vi "SISE-Monitor100.vi"() -> ()   [LabVIEW 2024]
uses:
  SubVIs-SISE-Monitor100/Control-IonFlux.ctl
  <vilib>/DAQmx/read.llb/DAQmx Read (Analog 2D DBL NChan NSamp).vi
  <vilib>/Instr/_visa.llb/VISA Configure Serial Port (Instr).vi
  <vilib>/DAQmx/create/channels.llb/DAQmx Create Channel (AI-Voltage-Basic).vi
  <vilib>/DAQmx/miscellaneous.llb/DAQmx Fill In Error Info.vi
  <vilib>/Analysis/NI_AALPro.lvlib
panel:
  out "Lesepuffer":string
  out "Registerkarte":enum32{"Start", "Record", "Stop"}(tab)
  out "Output V ch 2":bool
  in  "V channel 2":bool
  out "Output V ch 1":bool
  in  "V channel 1":bool
  out "SISE channel 1":bool
  out "Output SISE ch 2":bool
  in  "SISE channel 2":bool
  out "slow":bool
  in  "Scan angle (degrees)":dbl(slide) scale=0.0..90.0
  out "?":dbl
  in  "VISA res. name":refnum<visa-resource-name> caption="VISA-Ressourcenname"
  in  "Start measurement":bool
  out "Data File":bool
  out "Ind. Channel In":bool
  in  "Data file":path
  out "Ind. Channel Out":bool
  out "?":dbl
  out "Record period (round at 5s)":dbl
  in  "Scan distance (µm)":dbl(slide)=50.0 scale=0.0..100.0
  in  "Record period (single track, s)":dbl(slide)=10.112359550561797 scale=0.0..60.0 scale format="%#_2f"
  in  "Manipulator Speed":bool
  out "fast":bool
  in  "Channels In":tag
  in  "Position of manipulator":bool
  out "right":bool
  out "left":bool
  in  "TC 3":T1(tab)
  in  "Range limit\nS1.1 (mV)":dbl(slide)=200.0 min=0.0 max=600.0 scale=0.2..600.0
  in  "Base line\nS1.1 (mV)":dbl(slide) scale=-300.0..300.0
  in  "Range limit\nS1.2 mV":dbl(slide)=30.0 scale=0.1..30.0
  in  "Base line \nS1.2 (mV)":dbl(slide) scale=-15.0..15.0
  out "dV-SISE channel 1":cluster{dbl[], dbl[]}[](graph)
  out "V-SISE channel 1":cluster{dbl[], dbl[]}[](graph)
  out "V-SISE channel 2":cluster{dbl[], dbl[]}[](graph)
  out "dV-SISE channel 2":cluster{dbl[], dbl[]}[](graph)
  in  "Range limit\nS2.1 (mV)":dbl(slide)=200.0 min=0.0 max=600.0 scale=0.2..600.0
  in  "Base line\nS2.1 (mV)":dbl(slide) scale=-300.0..300.0
  in  "Base line \nS2.2 (mV)":dbl(slide) scale=-15.0..15.0
  in  "Range limit\nS2.2 (mV)":dbl(slide)=30.0 scale=0.1..30.0
  out "Voltage channel 1":cluster{dbl[], dbl[]}[](graph)
  in  "Base line\nV1 (V)":dbl(slide) scale=-10.0..10.0
  in  "Range limit\nV1 (V)":dbl(slide)=24.63054187192118 min=0.0 max=600.0 scale=0.0..25.0
  in  "Base line\nV2 (V)":dbl(slide) scale=-10.0..10.0
  in  "Range limit\nV2 (V)":dbl(slide)=24.63054187192118 min=0.0 max=600.0 scale=0.0..25.0
  out "Voltage channel 2":cluster{dbl[], dbl[]}[](graph)
  out "V channel #2":bool
  out "V channel #1":bool
  out "SISE channel #2":bool
  out "SISE channel #1":bool
  in  "?":T2(tab)
  out "Vprobe SISE 1":cluster{dbl[], dbl[]}[](graph)
  out "Vprobe SISE 2":cluster{dbl[], dbl[]}[](graph)
  out "Vprobe V 1":cluster{dbl[], dbl[]}[](graph)
  out "Vprobe V 2":cluster{dbl[], dbl[]}[](graph)
  in  "Enable change position 0":bool
  out "Raw data file":path
  in  "Stop measurent":bool
  out "Position probe":cluster{dbl[], dbl[]}[](graph)
  in  "Add Mark":bool
  in  "Event Mark":string
  out "Stop recording":bool
  out "String":string
  out "E-mark on":T3
  out "?":string
  in  "Bildlaufleiste":i32(c297)
  in  "Start fit (% of rec. period)":dbl(slide)=50.0 scale=0.0..100.0
  in  "?":enum32{"dV SISE 1", "dV SISE 2"}(tab)
  out "deltaV SISE 1":cluster{dbl[], "Best Linear Fit":dbl[]}[](graph)
  out "deltaV SISE 2":cluster{dbl[], "Best Linear Fit":dbl[]}[](graph)
  in  "Zoom from start":dbl(slide) scale=0.0..100.0
  in  "Zoom from end":dbl(slide)=100.0 scale=0.0..100.0
  in  "Stop programm":bool
  in  "New measurement":bool
  out "Stop recording 2":bool
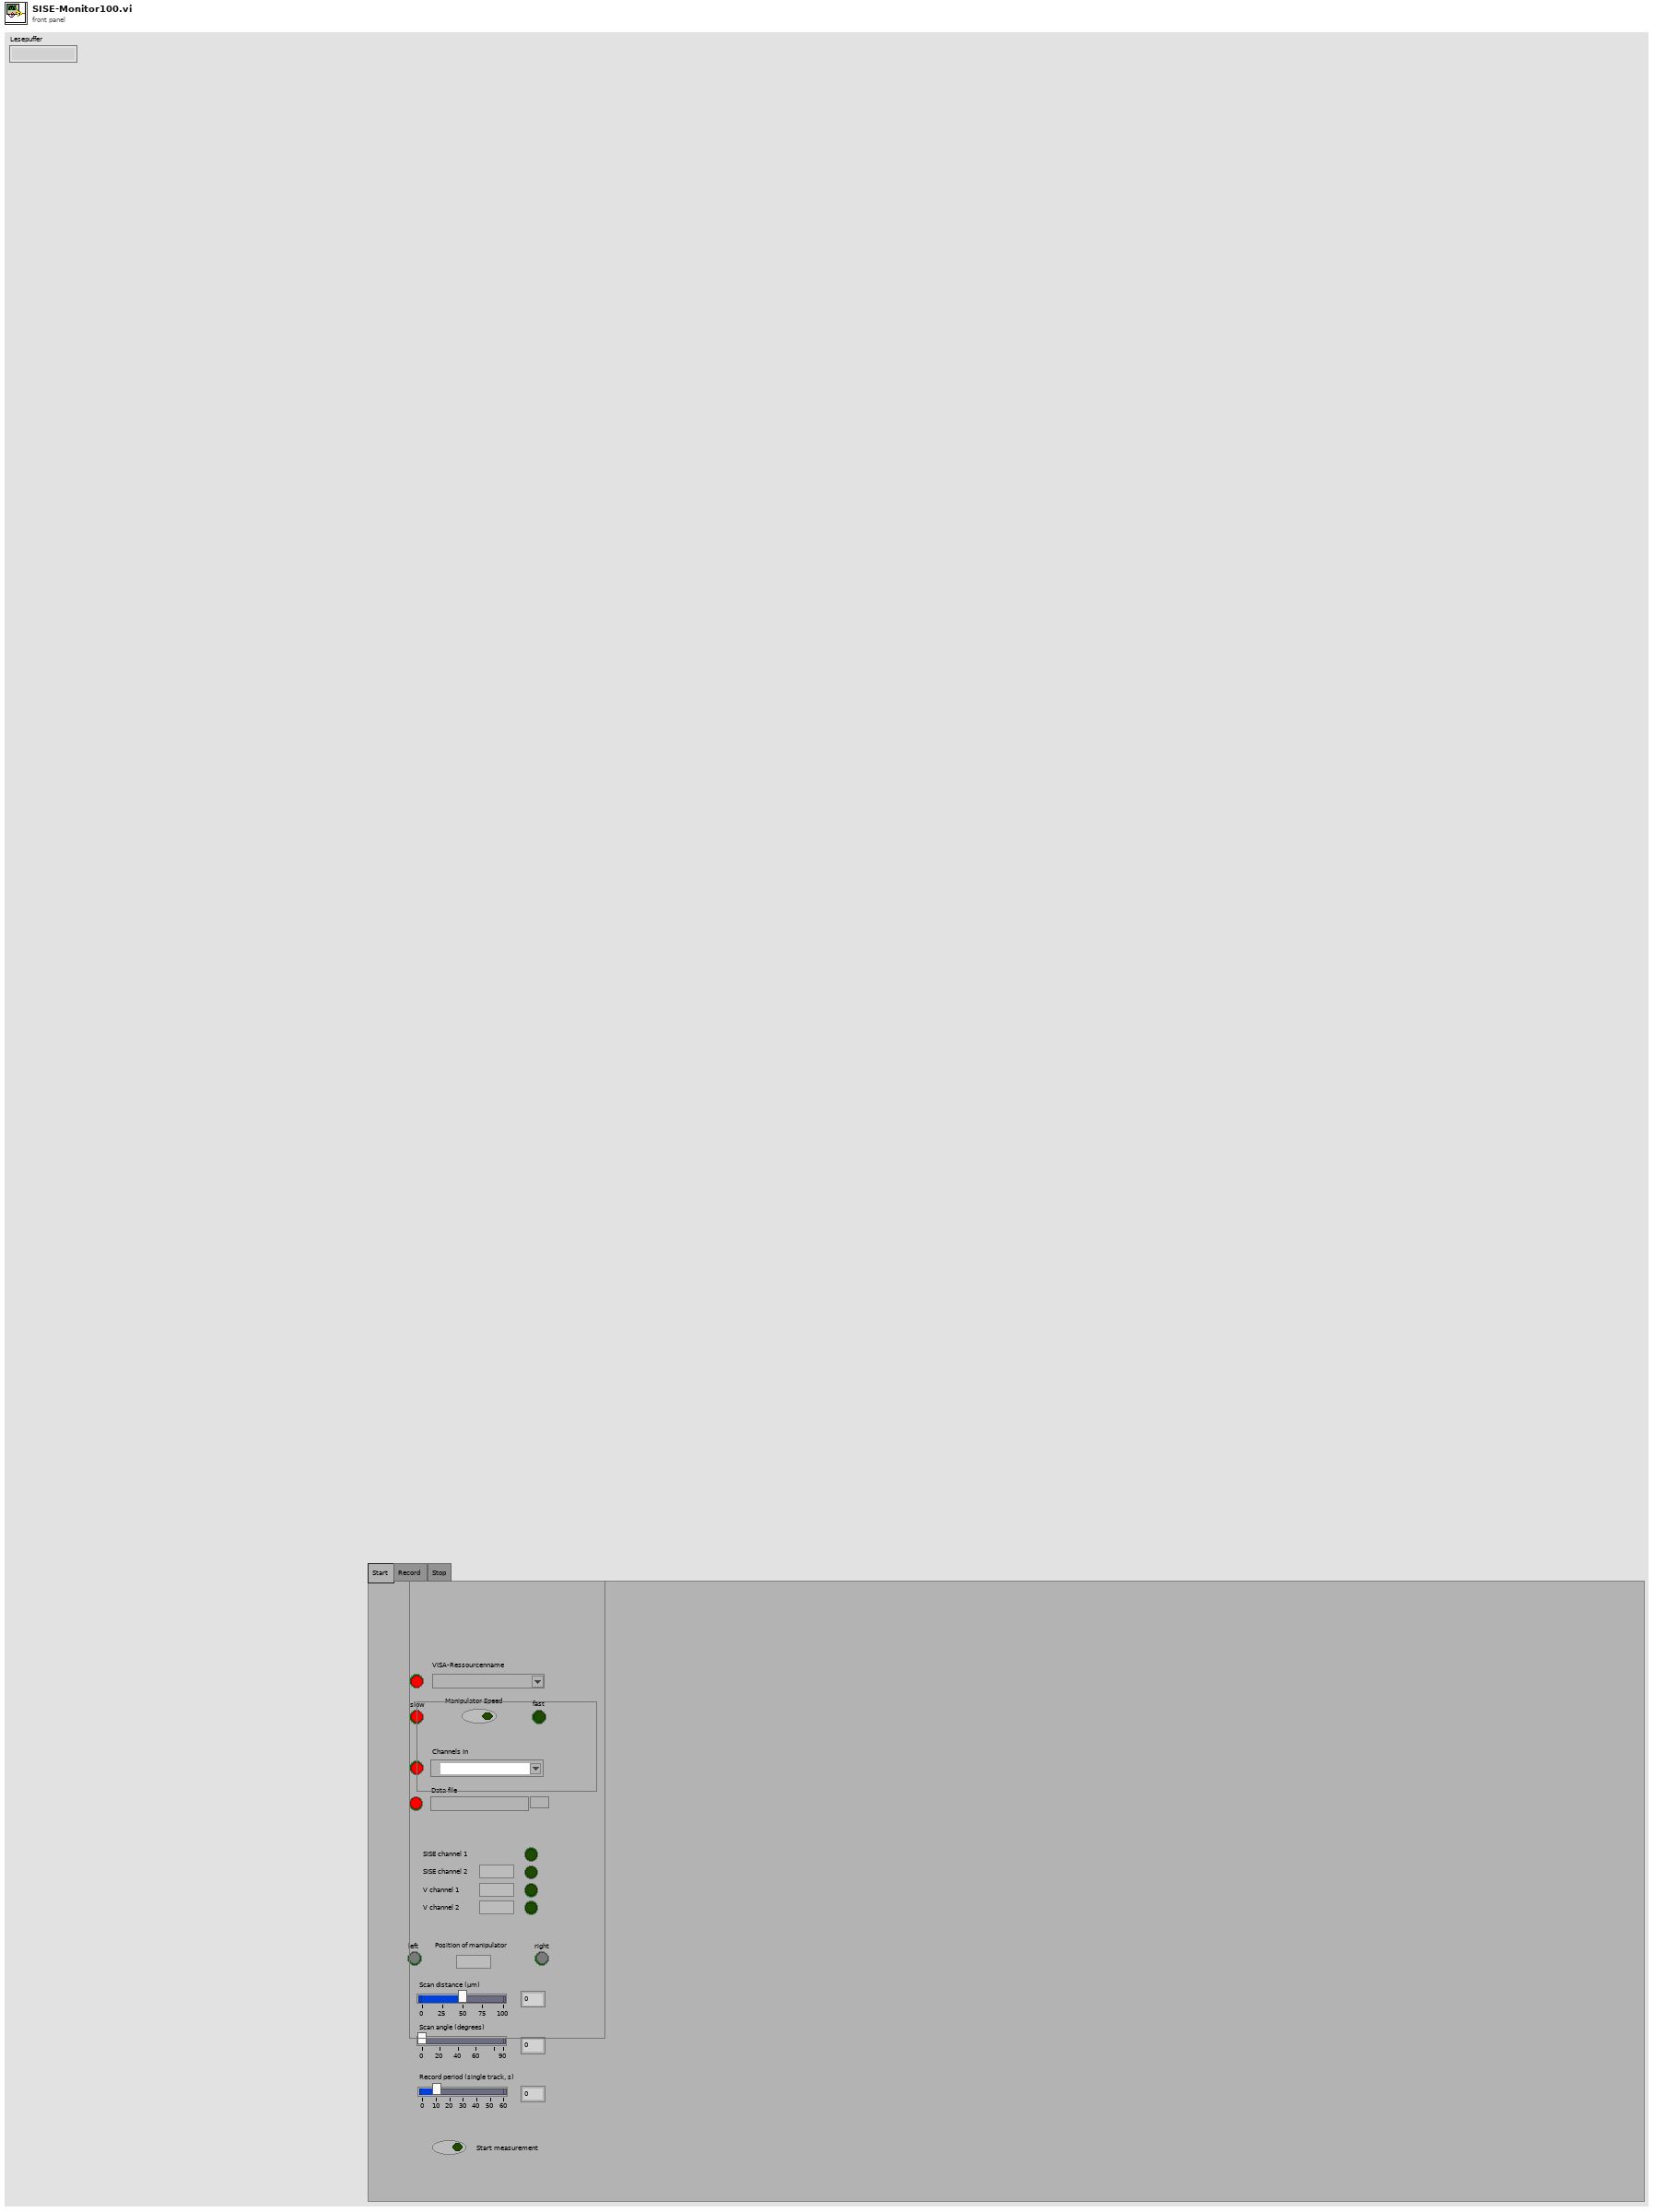
[diagram p1: front panel]
types:
  T1 = enum32{"SISE channel #1", "SISE channel #2", "V channel #1", "V channel #2"}
  T2 = enum32{"SISE chan #1", "SISE chan #2", "V chan #1", "V chan #2"}
  T3 = typedef "Control-IonFlux.ctl" = bool
  T4 = cluster{"refnum out":refnum<file>, "status":bool, "code":i32, "source":string}
  T5 = cluster{"task out":refnum<k21>, "status":bool, "code":i32, "source":string}
  T6 = enum16{"open", "replace", "create", "open or create", "replace or create", "replace or create with confirmation"}
  T7 = cluster{"refnum":refnum<file>, "status":bool, "code":i32, "source":string}
  T8 = cluster{dbl[], dbl[], "Best Linear Fit":dbl[], dbl[], dbl[]}
  T9 = cluster{"Array (Ausgang)":dbl[], "Array (Ausgang)":dbl[]}
  T10 = cluster{"Array (Ausgang)":dbl[], "Array (Ausgang)":dbl[]}[]
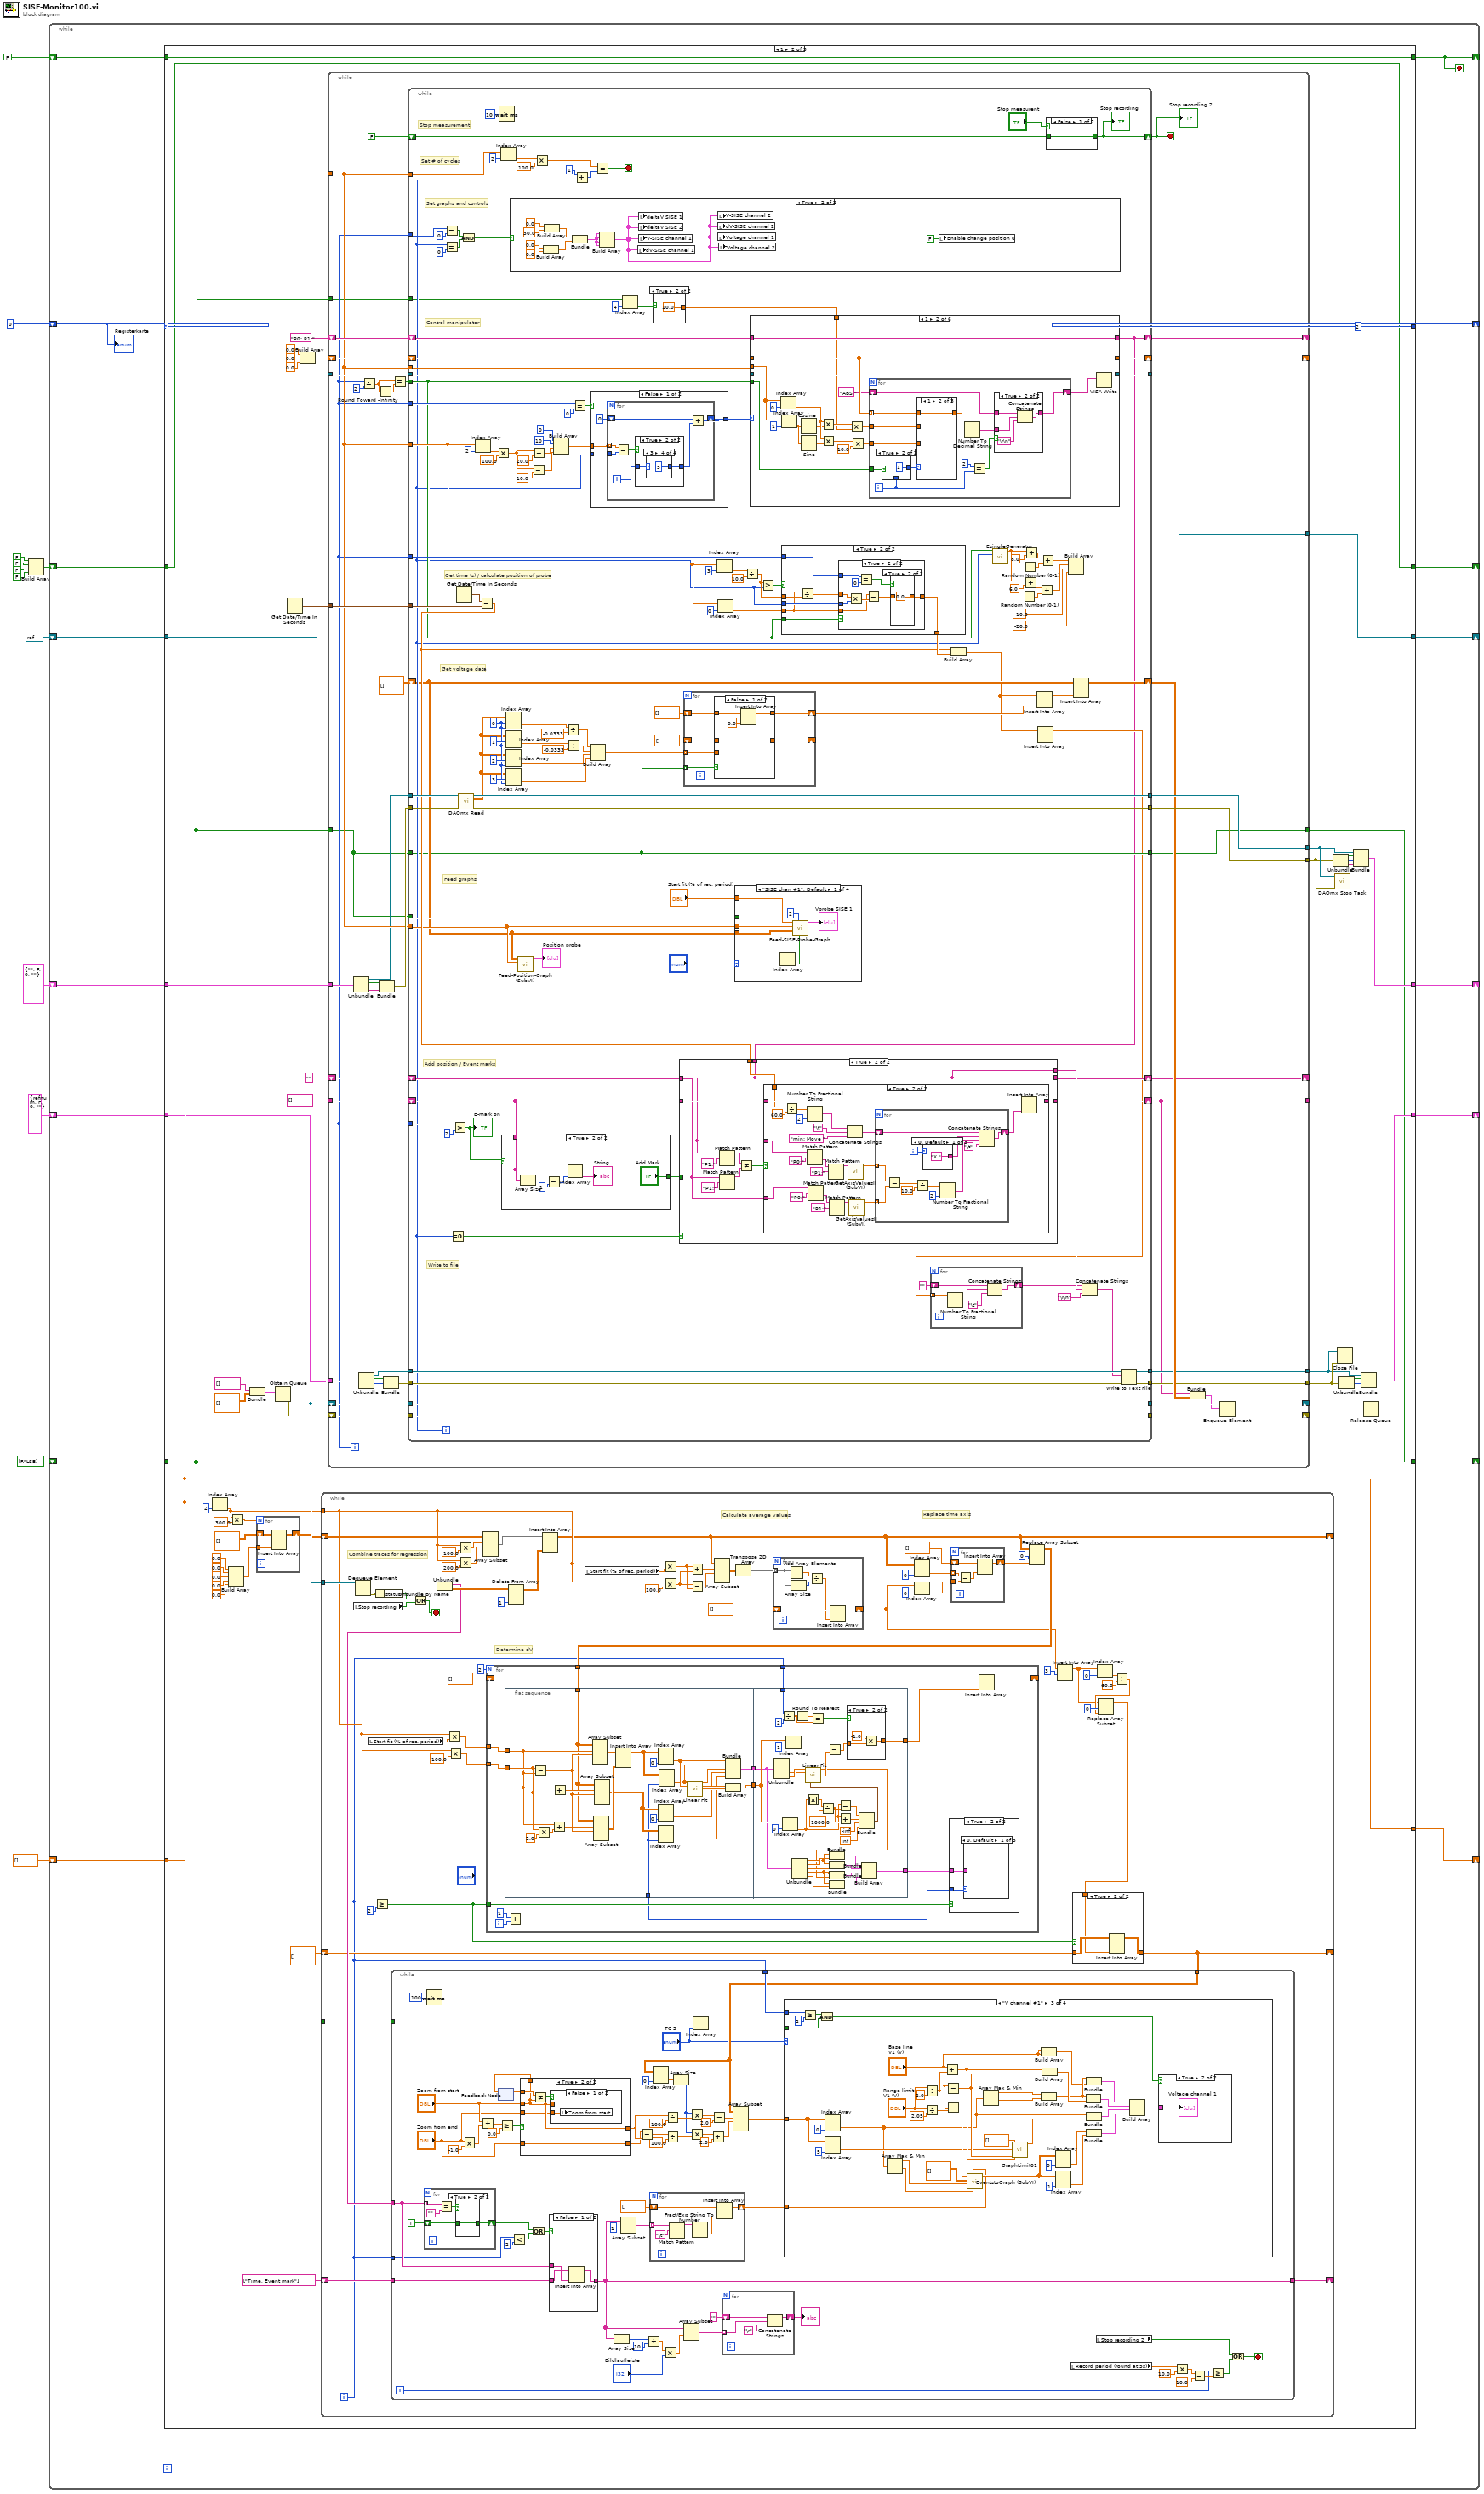
[diagram p0: block diagram]
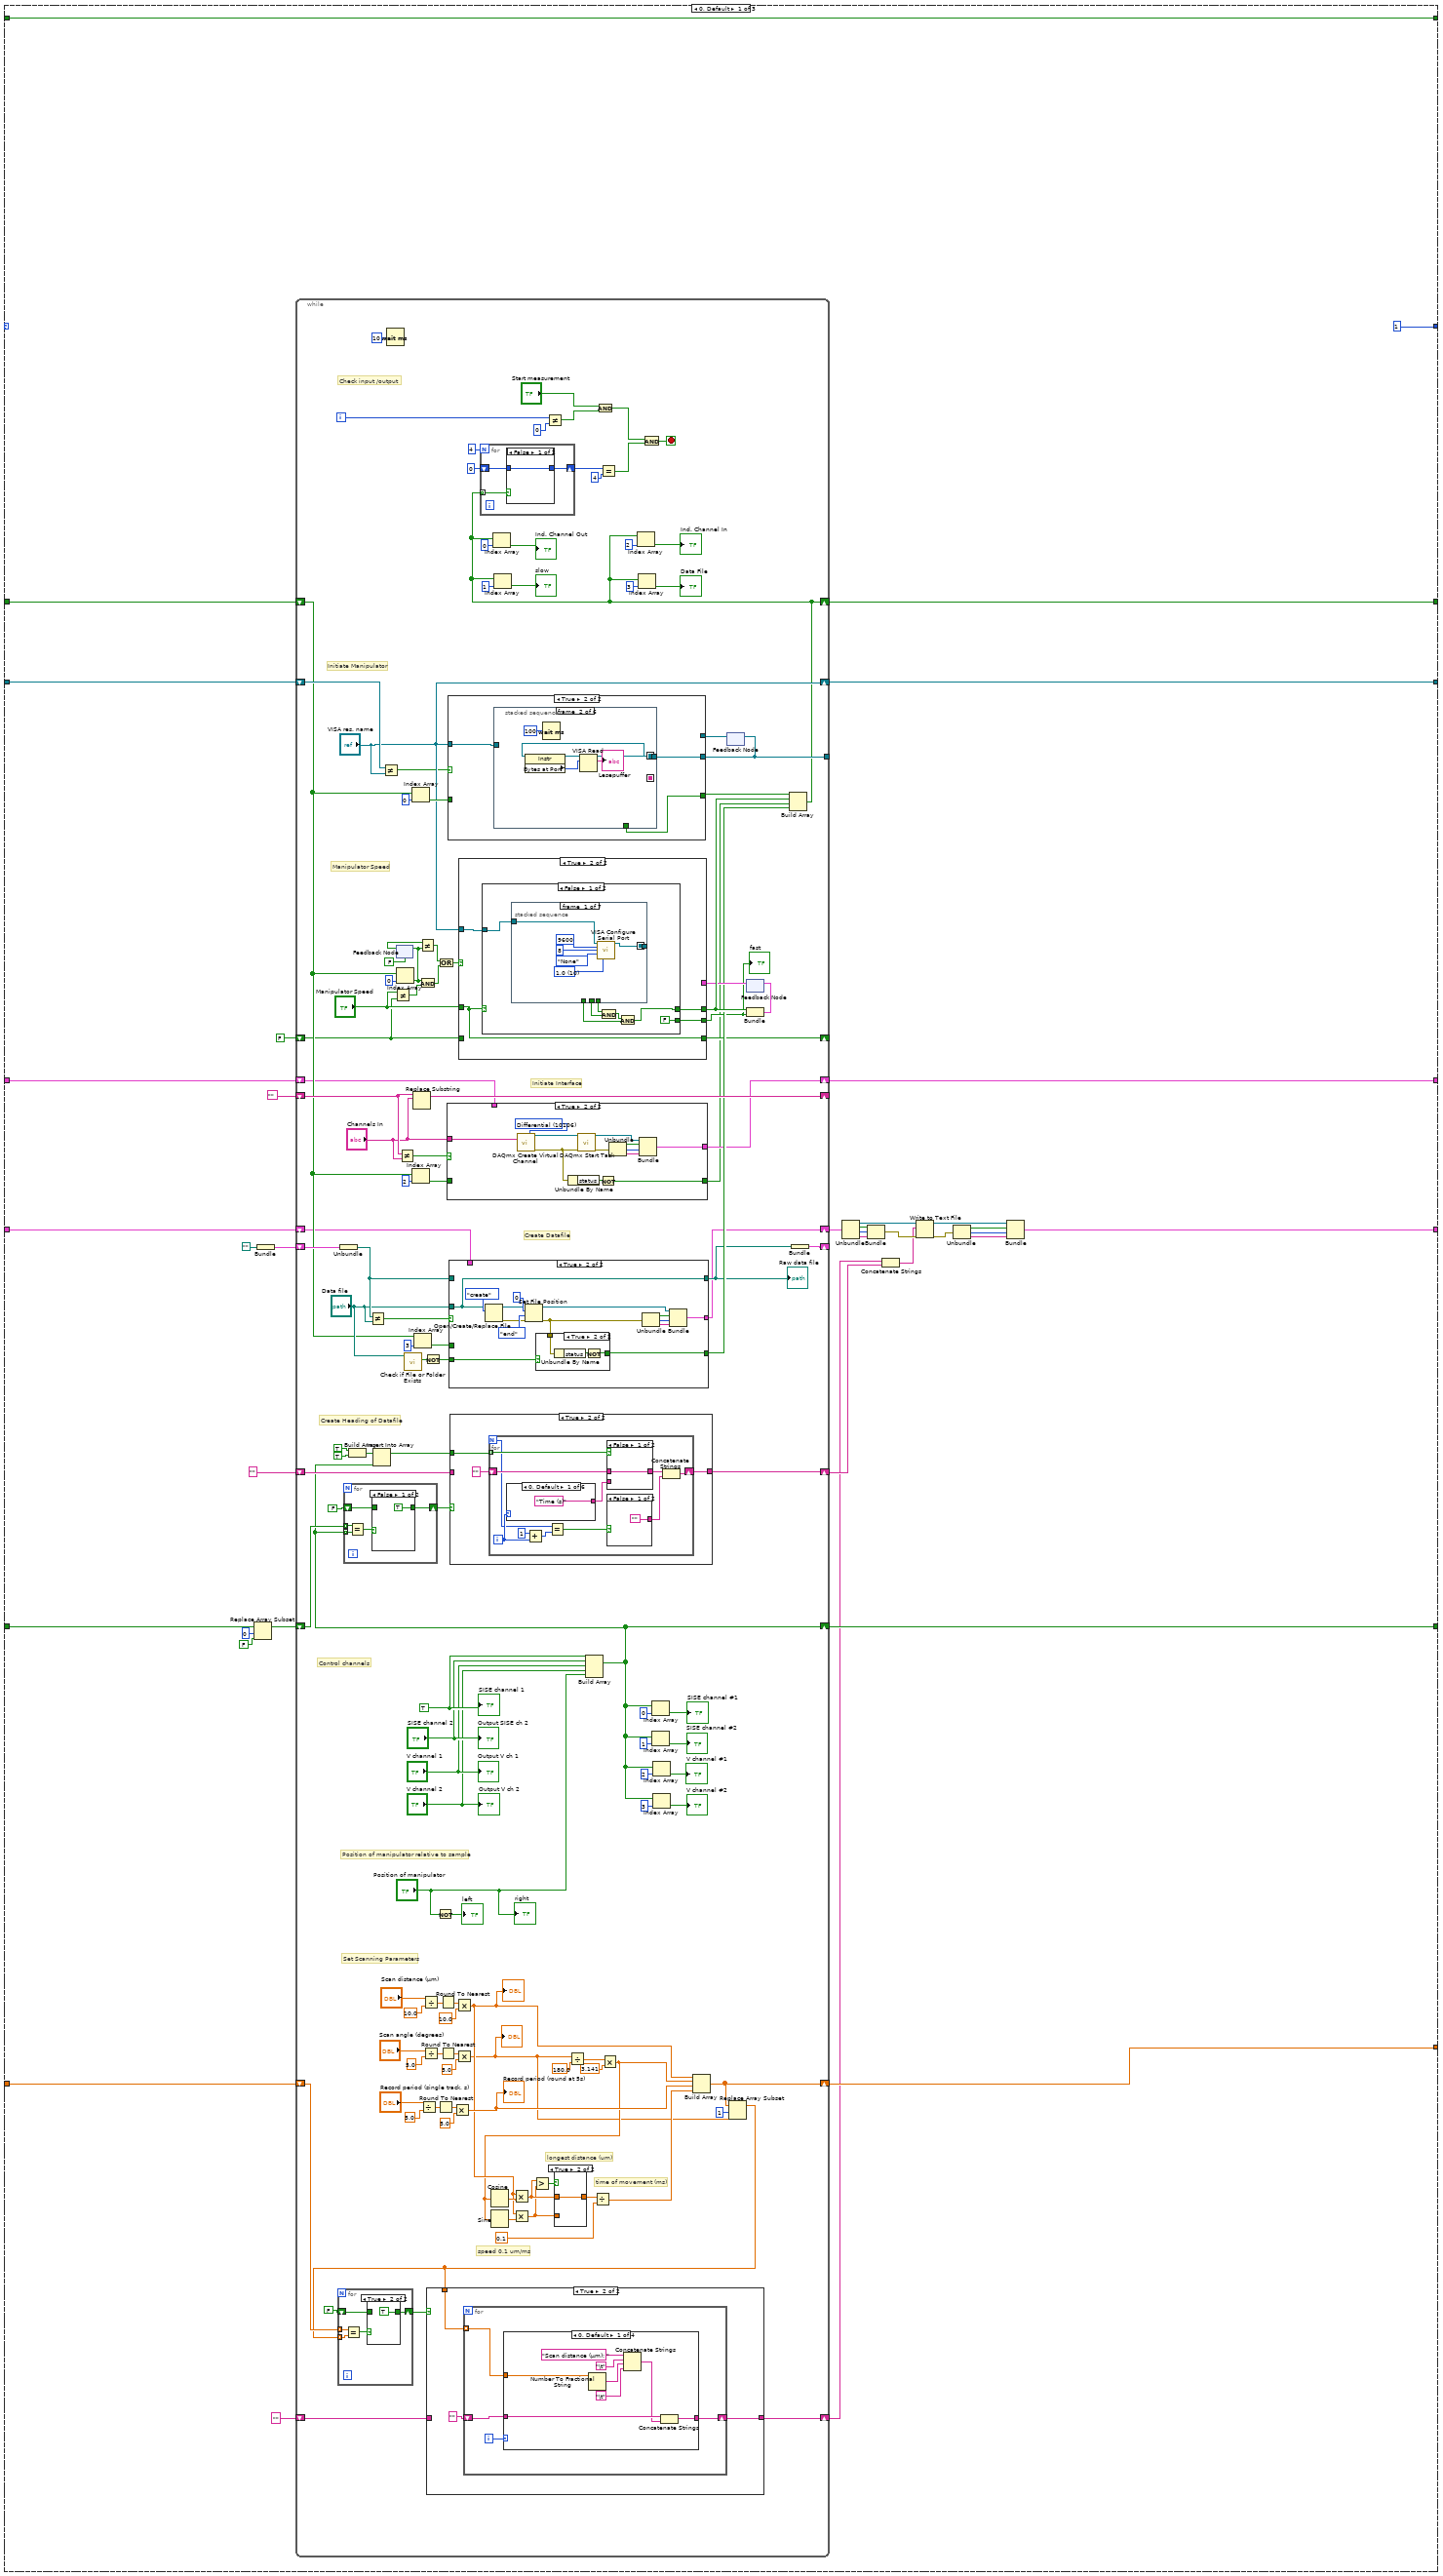
[diagram p2: hidden frame]
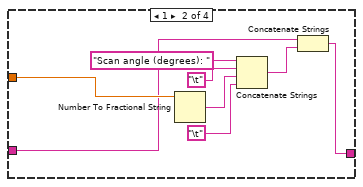
[diagram p4: hidden frame]
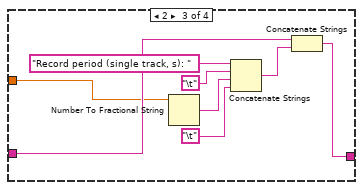
[diagram p5: hidden frame]
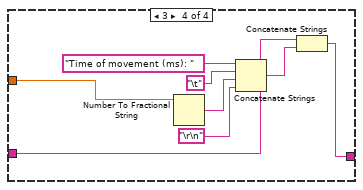
[diagram p6: hidden frame]
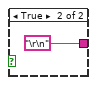
[diagram p10: hidden frame]
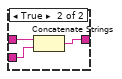
[diagram p11: hidden frame]
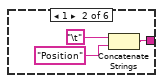
[diagram p12: hidden frame]
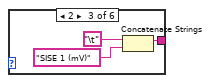
[diagram p13: hidden frame]
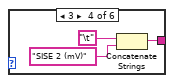
[diagram p14: hidden frame]
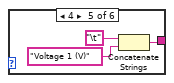
[diagram p15: hidden frame]
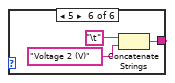
[diagram p16: hidden frame]
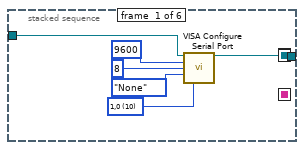
[diagram p18: hidden frame]
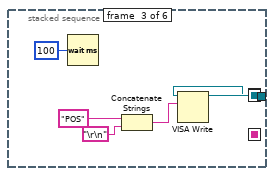
[diagram p19: hidden frame]
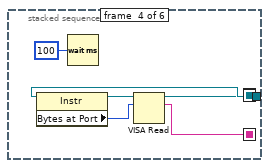
[diagram p20: hidden frame]
diagram:
  n1 = Build Array(FALSE, FALSE, FALSE, FALSE) -> (w1:bool[])
  n2 = while {
    shift-right: [w28] -> _
    shift-left: 0 -> [w27]
    shift-right: [w25] -> _
    shift-left: refnum<visa-resource-name> refnum ("VISA res. name") -> [w26]
    shift-right: [w23] -> _
    shift-left: T5 {"task out"="", "status"=FALSE, "code"=0, "source"=""} -> [w24]
    shift-right: [w19] -> _
    shift-left: T4 {"refnum out"=refnum, "status"=FALSE, "code"=0, "source"=""} -> [w20]
    shift-right: [w22] -> _
    shift-left: dbl[] [] -> [w21]
    shift-right: [w18] -> _
    shift-left: bool[] [FALSE] -> [w17]
    shift-right: [w15] -> _
    shift-left: FALSE -> [w16]
    shift-right: [w13] -> _
    shift-left: w1 -> [w14]
    stop <- w15 stop-if-true
    n3 = case shown="1" w27 {
      tunnel: [1 2 0] -> w28
      tunnel: w26 -> [w60 w553 w1602]
      tunnel: [w59 w552 w1602] -> w25
      tunnel: w24 -> [w58 w551 w1601]
      tunnel: [w57 w547 w1601] -> w23
      tunnel: [w40 w526 w1599] -> w19
      tunnel: w20 -> [w56 w530 w1599]
      tunnel: [w55 w540 w1600] -> w22
      tunnel: w21 -> [w54 w540 w1600]
      tunnel: w17 -> [w31 w510 w1598]
      tunnel: [w53 w523 w1598] -> w18
      tunnel: w16 -> [w39 w516 w1597]
      tunnel: [w39 w516 w1596] -> w15
      tunnel: w14 -> [w33 w515 w1595]
      tunnel: [w38 w515 w1595] -> w13
      frame 0, Default {
        n4 = Replace Array Subset(array=w31, new element=FALSE ("Neues Element/Teil-Array"), index=0 ("Index")) -> (w32:bool[])
        n5 = Bundle(path "") -> (w61:cluster{path})  [unwired: 1 in]
        n6 = while {
          shift-right: ["VISA res. name"] -> w59
          shift-left: w60 -> [w183]
          shift-right: [w90] -> w38
          shift-left: w33 -> [w137]
          tunnel: [w139] -> _
          shift-right: [w178] -> _
          shift-left: "" -> [w177]
          shift-right: [w168] -> _
          shift-left: w61 -> [w170]
          shift-right: [w119] -> _
          shift-left: FALSE -> [w134]
          shift-right: [w116] -> w57
          shift-left: w58 -> [w117]
          shift-right: [w114] -> w51
          shift-left: w56 -> [w113]
          shift-right: [w73] -> w55
          shift-left: w54 -> [w77]
          shift-right: [w66] -> w53
          shift-left: w32 -> [w85]
          shift-right: [w87] -> w36
          shift-left: "" -> [w86]
          shift-right: [w79] -> w35
          shift-left: "" -> [w75]
          i -> [w81]
          stop <- w83 stop-if-true
          w109 = TRUE
          # "Position of manipulator relative to sample"
          # "Set Scanning Parameters"
          # "Control channels"
          # "Create Heading of Datafile"
          # "Create Datafile"
          # "Initiate Interface"
          # "Manipulator Speed"
          # "Initiate Manipulator"
          # "Check input /output"
          # "speed 0.1 um/ms"
          # "longest distance (um)"
          # "time of movement (ms)"
          n7 = Unbundle(w170) -> (w169:path)
          n8 = Build Array(TRUE, TRUE) -> (w94:bool[])
          n9 = Not Equal?(x=w169, y="Data file") -> (x != y?=w93:bool)
          n10 = Not Equal?(x=w183, y="VISA res. name") -> (x != y?=w80:bool)
          n11 = Wait (ms)(milliseconds to wait=u32 10) -> ()  [unwired: 1 out]
          n12 = Not Equal?(x="Manipulator Speed", y=w134) -> (x != y?=w136:bool)
          n13 = feedback #1(FALSE) -> (w131:bool)
          n14 = Index Array(array=w137, index=0 ("Index")) -> (element=w132:bool)
          n15 = feedback-in #1(w132) -> ()
          n16 = Not Equal?(x=w177, y="Channels In") -> (x != y?=w180:bool)
          n17 = call <vilib>:"Check if File or Folder Exists.vi"("path"="Data file") -> ("file or folder exists?"=w174:bool)  [unwired: 8 in, 2 out]
          n18 = Index Array(array=w137, index=2 ("Index")) -> (element=w179:bool)
          n19 = Index Array(array=w137, index=0 ("Index")) -> (element=w143:bool)
          n20 = Replace Substring(4:"Channels In", 5:w177) -> (1:w178:string)  [unwired: 2 in, 1 out]
          n21 = Index Array(array=w137, index=3 ("Index")) -> (element=w171:bool)
          n22 = Not Equal?(x=w131, y=w132) -> (x != y?=w130:bool)
          n23 = And(x=w132, y=w136) -> (x .and. y?=w128:bool)
          n24 = Divide(x="Record period (single track, s)", y=5.0) -> (x/y=w184:dbl)
          n25 = Divide(x="Scan distance (µm)", y=10.0) -> (x/y=w191:dbl)
          n26 = Divide(x="Scan angle (degrees)", y=5.0) -> (x/y=w158:dbl)
          n27 = Not(x=w174) -> (.not. x?=w166:bool)
          n28 = Not(x="Position of manipulator") -> (.not. x?=→"left":bool)
          n29 = Round To Nearest(number=w184) -> (nearest integer value=w187:dbl)
          n30 = Or(x=w130, y=w128) -> (x .or. y?=w129:bool)
          n31 = Round To Nearest(number=w191) -> (nearest integer value=w190:dbl)
          n32 = Round To Nearest(number=w158) -> (nearest integer value=w157:dbl)
          n33 = case shown="True" w180 {
            tunnel: w179 -> [w367 _]
            tunnel: [w367 w378] -> w69
            tunnel: "Channels In" -> [_ w369]
            tunnel: w117 -> [w366 _]
            tunnel: [w366 w372] -> w116
            frame False {
            }
            frame True {
              w368 = 10106 items=["Default"=-1, "RSE"=10083, "NRSE"=10078, "Differential"=10106, "Pseudodifferential"=12529] ("input terminal configuration")
              n34 = call-poly <vilib>:"DAQmx Create Virtual Channel.vi"("input terminal configuration"=w368, "physical channels"=w369) -> ("task out"=w371:refnum<k21>, "error out"=w370:errorcluster)  [unwired: 12 in]
              n35 = Unbundle By Name(w370) -> ("status"=w379:bool)
              n36 = call <vilib>:"DAQmx Start Task.vi"("task/channels in"=w371, "error in"=w370) -> ("task out"=w373:refnum<k21>, "error out"=w377:errorcluster)  [unwired: 12 in]
              n37 = Not(x=w379) -> (.not. x?=w378:bool)
              n38 = Unbundle(w377) -> ("status"=w374:bool, "code"=w375:i32, "source"=w376:string)
              n39 = Bundle("task out"=w373, "status"=w374, "code"=w375, "source"=w376) -> (w372:T5)  [unwired: 1 in]
            }
          }
          n40 = case shown="True" w93 {
            tunnel: "Data file" -> [_ w355]
            tunnel: [w347 w356] -> w120
            tunnel: w171 -> [w347 _]
            tunnel: w169 -> [w346 _]
            tunnel: [w346 w355] -> w115
            tunnel: w166 -> [_ w354]
            tunnel: [w345 w350] -> w114
            tunnel: w113 -> [w345 _]
            frame False {
            }
            frame True {
              n41 = Open/Create/Replace File(file path (use dialog)=w355, operation (0:open)=T6."create") -> (refnum out=w359:refnum<file>, error out=w358:errorcluster)  [unwired: 4 in, 1 out]
              n42 = Set File Position(offset (in bytes) (0)=i64 0, refnum=w359, from (0:start)=enum16{"start", "end", "current"}."end", error in=w358) -> (refnum out=w348:refnum<file>, error out=w349:errorcluster)
              n43 = case shown="True" w354 {
                tunnel: [FALSE w364] -> w356
                tunnel: w349 -> [_ w363]
                frame False {
                }
                frame True {
                  n44 = Unbundle By Name(w363) -> ("status"=w365:bool)
                  n45 = Not(x=w365) -> (.not. x?=w364:bool)
                }
              }
              n46 = Unbundle(w349) -> ("status"=w353:bool, "code"=w352:i32, "source"=w351:string)
              n47 = Bundle("refnum"=w348, "status"=w353, "code"=w352, "source"=w351) -> (w350:T7)  [unwired: 1 in]
            }
          }
          "Raw data file" <- w115
          n48 = Multiply(x=w187, y=5.0) -> (x*y=w153:dbl)
          "Record period (round at 5s)" <- w153
          n49 = Multiply(x=w190, y=10.0) -> (x*y=w147:dbl)
          "?" <- w147
          n50 = Multiply(x=w157, y=5.0) -> (x*y=w71:dbl)
          "?" <- w71
          n51 = Not Equal?(x=w81, y=0) -> (x != y?=w163:bool)
          n52 = Divide(x=w71, y=180.0) -> (x/y=w110:dbl)
          n53 = Build Array(w109, "SISE channel 2", "V channel 1", "V channel 2", "Position of manipulator") -> (w66:bool[])
          n54 = for {
            tunnel: w85 -> [w246] mode=indexing
            tunnel: w66 -> [w245] mode=indexing
            shift-right: [w242] -> w82
            shift-left: FALSE -> [w243]
            n55 = Equal?(x=w246, y=w245) -> (x = y?=w244:bool)
            n56 = case shown="False" w244 {
              tunnel: w243 -> [_ w248]
              tunnel: [TRUE w248] -> w242
              frame False {
              }
              frame True {
              }
            }
          }
          n57 = Insert Into Array(array=w94, new element=w66) -> (w88:bool[])  [unwired: 1 in]
          n58 = case shown="True" w82 {
            tunnel: w88 -> [_ w251]
            tunnel: [w249 w250] -> w87
            tunnel: w86 -> [w249 _]
            frame False {
            }
            frame True {
              n59 = for {
                N -> [w255]
                shift-right: [w260] -> w250
                shift-left: "" -> [w263]
                tunnel: w251 -> [w261] mode=indexing
                i -> [w258]
                n60 = case shown="0, Default" w258 {
                  tunnel: ["Time (s)" w273 w276 w279 w282 w285] -> w262
                  frame 0, Default {
                  }
                  frame 1 {
                    n61 = Concatenate Strings("\t", "Position") -> (w273:string)
                  }
                  frame 2 {
                    n62 = Concatenate Strings("\t", "SISE 1 (mV)") -> (w276:string)
                  }
                  frame 3 {
                    n63 = Concatenate Strings("\t", "SISE 2 (mV)") -> (w279:string)
                  }
                  frame 4 {
                    n64 = Concatenate Strings("\t", "Voltage 1 (V)") -> (w282:string)
                  }
                  frame 5 {
                    n65 = Concatenate Strings("\t", "Voltage 2 (V)") -> (w285:string)
                  }
                }
                n66 = Add(x=1, y=w258) -> (x+y=w256:i32)
                n67 = Equal?(x=w255, y=w256) -> (x = y?=w254:bool)
                n68 = case shown="False" w261 {
                  tunnel: w263 -> [w266 w269]
                  tunnel: [w266 w268] -> w259
                  tunnel: w262 -> [_ w267]
                  frame False {
                  }
                  frame True {
                    n69 = Concatenate Strings(w269, w267) -> (w268:string)
                  }
                }
                n70 = case shown="False" w254 {
                  tunnel: ["" "\r\n"] -> w253
                  frame False {
                  }
                  frame True {
                  }
                }
                n71 = Concatenate Strings(w259, w253) -> (w260:string)
              }
            }
          }
          n72 = And(x="Start measurement", y=w163) -> (x .and. y?=w89:bool)
          n73 = Multiply(x=w110, y=3.141) -> (x*y=w74:dbl)
          n74 = Cosine(x=w74) -> (cos(x)=w152:dbl)
          n75 = Sine(x=w74) -> (sin(x)=w151:dbl)
          n76 = Multiply(x=w147, y=w152) -> (x*y=w150:dbl)
          n77 = Multiply(x=w147, y=w151) -> (x*y=w149:dbl)
          n78 = Greater?(x=w150, y=w149) -> (0:w148:bool)
          n79 = case shown="True" w148 {
            tunnel: w150 -> [_ w337]
            tunnel: w149 -> [w336 _]
            tunnel: [w336 w337] -> w146
            frame False {
            }
            frame True {
            }
          }
          n80 = Divide(x=w146, y=0.1) -> (x/y=w144:dbl)
          n81 = Index Array(array=w66, index=0 ("Index")) -> (element=→"SISE channel #1":bool)
          n82 = Index Array(array=w66, index=1 ("Index")) -> (element=→"SISE channel #2":bool)
          n83 = Index Array(array=w66, index=2 ("Index")) -> (element=→"V channel #1":bool)
          n84 = Index Array(array=w66, index=3 ("Index")) -> (element=→"V channel #2":bool)
          n85 = Build Array(w147, w74, w153, w144) -> (w73:dbl[])
          n86 = feedback #2() -> (w142:refnum<visa-resource-name>)  [unwired: 1 in]
          n87 = case shown="True" w80 {
            tunnel: w143 -> [w287 _]
            tunnel: [w287 w290] -> w127
            tunnel: "VISA res. name" -> [_ w289]
            tunnel: [w286 w288] -> w139
            tunnel: w142 -> [w286 _]
            frame False {
            }
            frame True {
              n88 = stacked-sequence {
                seq-local: [w291 _ _ _ _ _] -> [_ w298 _ _ _ _]
                seq-local: [_ w299 _ _ _ _] -> [_ _ w303 _ _ _]
                seq-local: [_ _ w304 _ _ _] -> [_ _ _ w311 _ _]
                seq-local: [_ _ _ w310 _ _] -> [_ _ _ _ w322 _]
                seq-local: [_ _ _ w309 _ _] -> [_ _ _ _ w316 _]
                seq-local: [_ _ _ _ w321 _] -> [_ _ _ _ _ w332]
                tunnel: w289 -> [w296 _ _ _ _ _]
                tunnel: [_ _ _ _ _ w331] -> w288
                tunnel: [_ _ _ _ _ w326] -> w290
                frame #0 {
                  w292 = u16 10 items=["1,0"=10, "1,5"=15, "2,0"=20] ("stop bits (10: 1 bit)")
                  n89 = call-poly "VISA Configure Serial Port"("VISA resource name"=w296, "baud rate (9600)"=u32 9600, "data bits (8)"=u16 8, "parity (0:none)"=enum16{"None", "Odd", "Even", "Mark", "Space"}."None", "stop bits (10: 1 bit)"=w292) -> ("VISA resource name out"=w291:refnum<visa-resource-name>)  [unwired: 9 in, 1 out]
                }
                frame #1 {
                  n90 = property class="Instr"(reference=w298) -> (reference out=w301:refnum<visa-resource-name>, "Bytes at Port"=w300:u32)  [unwired: 1 in, 1 out]
                  n91 = Wait (ms)(milliseconds to wait=u32 100) -> ()  [unwired: 1 out]
                  n92 = VISA Read(VISA resource name=w301, byte count=w300) -> (VISA resource name out=w299:refnum<visa-resource-name>, read buffer=→"Lesepuffer":string)  [unwired: 1 in, 2 out]
                }
                frame #2 {
                  n93 = Wait (ms)(milliseconds to wait=u32 100) -> ()  [unwired: 1 out]
                  n94 = Concatenate Strings("POS", "\r\n") -> (w305:string)
                  n95 = VISA Write(VISA resource name=w303, write buffer=w305) -> (VISA resource name out=w304:refnum<visa-resource-name>)  [unwired: 1 in, 2 out]
                }
                frame #3 {
                  n96 = property class="Instr"(reference=w311) -> (reference out=w312:refnum<visa-resource-name>, "Bytes at Port"=w313:u32)  [unwired: 1 in, 1 out]
                  n97 = Wait (ms)(milliseconds to wait=u32 100) -> ()  [unwired: 1 out]
                  n98 = VISA Read(VISA resource name=w312, byte count=w313) -> (VISA resource name out=w310:refnum<visa-resource-name>, read buffer=w309:string)  [unwired: 1 in, 2 out]
                }
                frame #4 {
                  n99 = String Length(string=w316) -> (length=w319:i32)
                  n100 = Subtract(x=w319, y=1) -> (x-y=w317:i32)
                  n101 = Wait (ms)(milliseconds to wait=u32 100) -> ()  [unwired: 1 out]
                  n102 = String Subset(string=w316, length (rest)=w317) -> (substring=w315:string)  [unwired: 1 in]
                  n103 = Concatenate Strings("ABS ", w315, "\r\n") -> (w323:string)
                  n104 = VISA Write(VISA resource name=w322, write buffer=w323) -> (VISA resource name out=w321:refnum<visa-resource-name>)  [unwired: 1 in, 2 out]
                }
                frame #5 {
                  n105 = property class="Instr"(reference=w332) -> (reference out=w333:refnum<visa-resource-name>, "Bytes at Port"=w334:u32)  [unwired: 1 in, 1 out]
                  n106 = Wait (ms)(milliseconds to wait=u32 100) -> ()  [unwired: 1 out]
                  n107 = VISA Read(VISA resource name=w333, byte count=w334) -> (VISA resource name out=w331:refnum<visa-resource-name>, read buffer=w327:string)  [unwired: 1 in, 2 out]
                  n108 = Concatenate Strings("A", "\r") -> (w330:string)
                  n109 = Equal?(x=w327, y=w330) -> (x = y?=w326:bool)
                }
              }
            }
          }
          n110 = feedback-in #2(w139) -> ()
          n111 = Replace Array Subset(array=w73, new element=w71, index=1 ("Index")) -> (w70:dbl[])
          n112 = for {
            shift-right: [w235] -> w76
            shift-left: FALSE -> [w236]
            tunnel: w77 -> [w239] mode=indexing
            tunnel: w70 -> [w238] mode=indexing
            n113 = Equal?(x=w239, y=w238) -> (x = y?=w237:bool)
            n114 = case shown="True" w237 {
              tunnel: w236 -> [w240 _]
              tunnel: [w240 TRUE] -> w235
              frame False {
              }
              frame True {
              }
            }
          }
          n115 = case shown="True" w76 {
            tunnel: [w195 w198] -> w79
            tunnel: w70 -> [_ w196]
            tunnel: w75 -> [w195 _]
            frame False {
            }
            frame True {
              n116 = for {
                tunnel: w196 -> [w199] mode=indexing
                shift-right: [w200] -> w198
                shift-left: "" -> [w201]
                i -> [w202]
                n117 = case shown="0, Default" w202 {
                  tunnel: [w210 w212 w222 w230] -> w200
                  tunnel: w201 -> [w209 w213 w221 w227]
                  tunnel: w199 -> [w205 w214 w220 w228]
                  frame 0, Default {
                    n118 = Number To Fractional String(number=w205) -> (F-format string=w204:string)  [unwired: 3 in]
                    n119 = Concatenate Strings("Scan distance (µm): ", "\t", w204, "\t") -> (w206:string)
                    n120 = Concatenate Strings(w209, w206) -> (w210:string)
                  }
                  frame 1 {
                    n121 = Number To Fractional String(number=w214) -> (F-format string=w218:string)  [unwired: 3 in]
                    n122 = Concatenate Strings("Scan angle (degrees): ", "\t", w218, "\t") -> (w211:string)
                    n123 = Concatenate Strings(w213, w211) -> (w212:string)
                  }
                  frame 2 {
                    n124 = Number To Fractional String(number=w220) -> (F-format string=w226:string)  [unwired: 3 in]
                    n125 = Concatenate Strings("Record period (single track, s): ", "\t", w226, "\t") -> (w219:string)
                    n126 = Concatenate Strings(w221, w219) -> (w222:string)
                  }
                  frame 3 {
                    n127 = Number To Fractional String(number=w228) -> (F-format string=w234:string)  [unwired: 3 in]
                    n128 = Concatenate Strings("Time of movement (ms): ", "\t", w234, "\r\n") -> (w229:string)
                    n129 = Concatenate Strings(w227, w229) -> (w230:string)
                  }
                }
              }
            }
          }
          n130 = feedback #3() -> (w124:cluster{bool, bool})  [unwired: 1 in]
          n131 = case shown="True" w129 {
            tunnel: "VISA res. name" -> [_ w387]
            tunnel: [w383 w386] -> w119
            tunnel: "Manipulator Speed" -> [_ w386]
            tunnel: w134 -> [w383 _]
            tunnel: [w380 w385] -> w126
            tunnel: [w381 w384] -> w91
            tunnel: w124 -> [w382 _]
            frame False {
              n132 = Unbundle(w382) -> (w380:bool, w381:bool)
            }
            frame True {
              n133 = case shown="False" w386 {
                tunnel: w387 -> [w394 w455]
                tunnel: [FALSE w449] -> w384
                tunnel: [w388 FALSE] -> w385
                frame False {
                  n134 = stacked-sequence {
                    seq-local: [w395 _ _ _ _ _ _] -> [_ w405 _ _ _ _ _]
                    seq-local: [_ w401 _ _ _ _ _] -> [_ _ w414 _ _ _ _]
                    seq-local: [_ _ w408 _ _ _ _] -> [_ _ _ w417 _ _ _]
                    seq-local: [_ _ _ w418 _ _ _] -> [_ _ _ _ w429 _ _]
                    seq-local: [_ _ _ _ w428 _ _] -> [_ _ _ _ _ w434 _]
                    seq-local: [_ _ _ _ _ w433 _] -> [_ _ _ _ _ _ w445]
                    tunnel: w394 -> [w400 _ _ _ _ _ _]
                    tunnel: [_ _ w407 _ _ _ _] -> w392
                    tunnel: [_ _ _ _ w423 _ _] -> w390
                    tunnel: [_ _ _ _ _ _ w444] -> _
                    tunnel: [_ _ _ _ _ _ w439] -> w391
                    frame #0 {
                      w396 = u16 10 items=["1,0"=10, "1,5"=15, "2,0"=20] ("stop bits (10: 1 bit)")
                      n135 = call-poly "VISA Configure Serial Port"("VISA resource name"=w400, "baud rate (9600)"=u32 9600, "data bits (8)"=u16 8, "parity (0:none)"=enum16{"None", "Odd", "Even", "Mark", "Space"}."None", "stop bits (10: 1 bit)"=w396) -> ("VISA resource name out"=w395:refnum<visa-resource-name>)  [unwired: 9 in, 1 out]
                    }
                    frame #1 {
                      n136 = Wait (ms)(milliseconds to wait=u32 100) -> ()  [unwired: 1 out]
                      n137 = Concatenate Strings("ACC 10", "\r\n") -> (w402:string)
                      n138 = VISA Write(VISA resource name=w405, write buffer=w402) -> (VISA resource name out=w401:refnum<visa-resource-name>)  [unwired: 1 in, 2 out]
                    }
                    frame #2 {
                      n139 = property class="Instr"(reference=w414) -> (reference out=w415:refnum<visa-resource-name>, "Bytes at Port"=w413:u32)  [unwired: 1 in, 1 out]
                      n140 = Wait (ms)(milliseconds to wait=u32 100) -> ()  [unwired: 1 out]
                      n141 = VISA Read(VISA resource name=w415, byte count=w413) -> (VISA resource name out=w408:refnum<visa-resource-name>, read buffer=w412:string)  [unwired: 1 in, 2 out]
                      n142 = Concatenate Strings("A", "\r") -> (w409:string)
                      n143 = Equal?(x=w412, y=w409) -> (x = y?=w407:bool)
                    }
                    frame #3 {
                      n144 = Wait (ms)(milliseconds to wait=u32 100) -> ()  [unwired: 1 out]
                      n145 = Concatenate Strings("FIRST 1000", "\r\n") -> (w419:string)
                      n146 = VISA Write(VISA resource name=w417, write buffer=w419) -> (VISA resource name out=w418:refnum<visa-resource-name>)  [unwired: 1 in, 2 out]
                    }
                    frame #4 {
                      n147 = property class="Instr"(reference=w429) -> (reference out=w430:refnum<visa-resource-name>, "Bytes at Port"=w431:u32)  [unwired: 1 in, 1 out]
                      n148 = Wait (ms)(milliseconds to wait=u32 100) -> ()  [unwired: 1 out]
                      n149 = Concatenate Strings("A", "\r") -> (w424:string)
                      n150 = VISA Read(VISA resource name=w430, byte count=w431) -> (VISA resource name out=w428:refnum<visa-resource-name>, read buffer=w427:string)  [unwired: 1 in, 2 out]
                      n151 = Equal?(x=w427, y=w424) -> (x = y?=w423:bool)
                    }
                    frame #5 {
                      n152 = Wait (ms)(milliseconds to wait=u32 100) -> ()  [unwired: 1 out]
                      n153 = Concatenate Strings("TOP 1000", "\r\n") -> (w435:string)
                      n154 = VISA Write(VISA resource name=w434, write buffer=w435) -> (VISA resource name out=w433:refnum<visa-resource-name>)  [unwired: 1 in, 2 out]
                    }
                    frame #6 {
                      n155 = property class="Instr"(reference=w445) -> (reference out=w446:refnum<visa-resource-name>, "Bytes at Port"=w447:u32)  [unwired: 1 in, 1 out]
                      n156 = Wait (ms)(milliseconds to wait=u32 100) -> ()  [unwired: 1 out]
                      n157 = VISA Read(VISA resource name=w446, byte count=w447) -> (VISA resource name out=w444:refnum<visa-resource-name>, read buffer=w440:string)  [unwired: 1 in, 2 out]
                      n158 = Concatenate Strings("A", "\r") -> (w443:string)
                      n159 = Equal?(x=w440, y=w443) -> (x = y?=w439:bool)
                    }
                  }
                  n160 = And(x=w392, y=w391) -> (x .and. y?=w393:bool)
                  n161 = And(x=w393, y=w390) -> (x .and. y?=w388:bool)
                }
                frame True {
                  n162 = stacked-sequence {
                    seq-local: [w456 _ _ _ _ _ _] -> [_ w466 _ _ _ _ _]
                    seq-local: [_ w462 _ _ _ _ _] -> [_ _ w475 _ _ _ _]
                    seq-local: [_ _ w469 _ _ _ _] -> [_ _ _ w478 _ _ _]
                    seq-local: [_ _ _ w479 _ _ _] -> [_ _ _ _ w490 _ _]
                    seq-local: [_ _ _ _ w489 _ _] -> [_ _ _ _ _ w495 _]
                    seq-local: [_ _ _ _ _ w494 _] -> [_ _ _ _ _ _ w506]
                    tunnel: w455 -> [w461 _ _ _ _ _ _]
                    tunnel: [_ _ w468 _ _ _ _] -> w453
                    tunnel: [_ _ _ _ w484 _ _] -> w451
                    tunnel: [_ _ _ _ _ _ w505] -> _
                    tunnel: [_ _ _ _ _ _ w500] -> w452
                    frame #0 {
                      w457 = u16 10 items=["1,0"=10, "1,5"=15, "2,0"=20] ("stop bits (10: 1 bit)")
                      n163 = call-poly "VISA Configure Serial Port"("VISA resource name"=w461, "baud rate (9600)"=u32 9600, "data bits (8)"=u16 8, "parity (0:none)"=enum16{"None", "Odd", "Even", "Mark", "Space"}."None", "stop bits (10: 1 bit)"=w457) -> ("VISA resource name out"=w456:refnum<visa-resource-name>)  [unwired: 9 in, 1 out]
                    }
                    frame #1 {
                      n164 = Wait (ms)(milliseconds to wait=u32 100) -> ()  [unwired: 1 out]
                      n165 = Concatenate Strings("ACC 500", "\r\n") -> (w463:string)
                      n166 = VISA Write(VISA resource name=w466, write buffer=w463) -> (VISA resource name out=w462:refnum<visa-resource-name>)  [unwired: 1 in, 2 out]
                    }
                    frame #2 {
                      n167 = property class="Instr"(reference=w475) -> (reference out=w476:refnum<visa-resource-name>, "Bytes at Port"=w474:u32)  [unwired: 1 in, 1 out]
                      n168 = Wait (ms)(milliseconds to wait=u32 100) -> ()  [unwired: 1 out]
                      n169 = VISA Read(VISA resource name=w476, byte count=w474) -> (VISA resource name out=w469:refnum<visa-resource-name>, read buffer=w473:string)  [unwired: 1 in, 2 out]
                      n170 = Concatenate Strings("A", "\r") -> (w470:string)
                      n171 = Equal?(x=w473, y=w470) -> (x = y?=w468:bool)
                    }
                    frame #3 {
                      n172 = Wait (ms)(milliseconds to wait=u32 100) -> ()  [unwired: 1 out]
                      n173 = Concatenate Strings("FIRST 1000", "\r\n") -> (w480:string)
                      n174 = VISA Write(VISA resource name=w478, write buffer=w480) -> (VISA resource name out=w479:refnum<visa-resource-name>)  [unwired: 1 in, 2 out]
                    }
                    frame #4 {
                      n175 = property class="Instr"(reference=w490) -> (reference out=w491:refnum<visa-resource-name>, "Bytes at Port"=w492:u32)  [unwired: 1 in, 1 out]
                      n176 = Wait (ms)(milliseconds to wait=u32 100) -> ()  [unwired: 1 out]
                      n177 = Concatenate Strings("A", "\r") -> (w485:string)
                      n178 = VISA Read(VISA resource name=w491, byte count=w492) -> (VISA resource name out=w489:refnum<visa-resource-name>, read buffer=w488:string)  [unwired: 1 in, 2 out]
                      n179 = Equal?(x=w488, y=w485) -> (x = y?=w484:bool)
                    }
                    frame #5 {
                      n180 = Wait (ms)(milliseconds to wait=u32 100) -> ()  [unwired: 1 out]
                      n181 = Concatenate Strings("TOP 30000", "\r\n") -> (w496:string)
                      n182 = VISA Write(VISA resource name=w495, write buffer=w496) -> (VISA resource name out=w494:refnum<visa-resource-name>)  [unwired: 1 in, 2 out]
                    }
                    frame #6 {
                      n183 = property class="Instr"(reference=w506) -> (reference out=w507:refnum<visa-resource-name>, "Bytes at Port"=w508:u32)  [unwired: 1 in, 1 out]
                      n184 = Wait (ms)(milliseconds to wait=u32 100) -> ()  [unwired: 1 out]
                      n185 = VISA Read(VISA resource name=w507, byte count=w508) -> (VISA resource name out=w505:refnum<visa-resource-name>, read buffer=w501:string)  [unwired: 1 in, 2 out]
                      n186 = Concatenate Strings("A", "\r") -> (w504:string)
                      n187 = Equal?(x=w501, y=w504) -> (x = y?=w500:bool)
                    }
                  }
                  n188 = And(x=w453, y=w452) -> (x .and. y?=w454:bool)
                  n189 = And(x=w454, y=w451) -> (x .and. y?=w449:bool)
                }
              }
            }
          }
          "fast" <- w91
          n190 = Bundle(w126, w91) -> (w125:cluster{bool, bool})  [unwired: 1 in]
          n191 = feedback-in #3(w125) -> ()
          n192 = Build Array(w127, w126, w69, w120) -> (w90:bool[])
          n193 = for {
            N: 4 -> [_]
            tunnel: w90 -> [w340] mode=indexing
            shift-right: [w338] -> w92
            shift-left: 0 -> [w339]
            n194 = case shown="False" w340 {
              tunnel: w339 -> [w341 w344]
              tunnel: [w341 w342] -> w338
              frame False {
              }
              frame True {
                n195 = Add(x=w344, y=1) -> (x+y=w342:i32)
              }
            }
          }
          n196 = Index Array(array=w90, index=0 ("Index")) -> (element=→"Ind. Channel Out":bool)
          n197 = Index Array(array=w90, index=1 ("Index")) -> (element=→"slow":bool)
          n198 = Equal?(x=w92, y=4) -> (x = y?=w159:bool)
          n199 = Index Array(array=w90, index=2 ("Index")) -> (element=→"Ind. Channel In":bool)
          n200 = Index Array(array=w90, index=3 ("Index")) -> (element=→"Data File":bool)
          n201 = And(x=w89, y=w159) -> (x .and. y?=w83:bool)
          n202 = Bundle("Data file"=w115) -> (w168:cluster{"Data file ":path})  [unwired: 1 in]
          "Output SISE ch 2" <- "SISE channel 2"
          "SISE channel 1" <- w109
          "Output V ch 1" <- "V channel 1"
          "Output V ch 2" <- "V channel 2"
          "right" <- "Position of manipulator"
        }
        n203 = Unbundle(w51) -> ("refnum out"=w46:refnum<file>, "status"=w50:bool, "code"=w49:i32, "source"=w48:string)
        n204 = Bundle("status"=w50, "code"=w49, "source"=w48) -> (w47:errorcluster)  [unwired: 1 in]
        n205 = Concatenate Strings(w35, w36) -> (w34:string)
        n206 = Write to Text File(file (use dialog)=w46, text=w34, error in=w47) -> (refnum out=w44:refnum<file>, error out=w45:errorcluster)  [unwired: 1 in, 1 out]
        n207 = Unbundle(w45) -> ("status"=w43:bool, "code"=w42:i32, "source"=w41:string)
        n208 = Bundle("refnum out"=w44, "status"=w43, "code"=w42, "source"=w41) -> (w40:T4)  [unwired: 1 in]
      }
      frame 1 {
        n209 = Index Array(array=w540, index=2 ("Index")) -> (element=w536:dbl)
        n210 = Build Array(0.0, 0.0, 0.0, 0.0, 0.0) -> (w517:dbl[])
        n211 = Multiply(x=w536, y=300.0 ("x")) -> (x*y=w541:dbl)
        n212 = Bundle(string[] [], dbl[][] []) -> (w533:cluster{string[], dbl[][]})  [unwired: 1 in]
        n213 = for {
          N: w541 -> [_]
          shift-right: [w563] -> w537
          shift-left: dbl[][] [] -> [w562]
          tunnel: w517 -> [w561]
          n214 = Insert Into Array(array=w562, new element=w561) -> (w563:dbl[][])  [unwired: 2 in]
        }
        n215 = Obtain Queue(element data type=w533) -> (queue out=w543:refnum<queue>, error out=w546:errorcluster)  [unwired: 4 in, 1 out]
        n216 = Get Date/Time In Seconds() -> (seconds since 1Jan1904=w559:timestamp)
        n217 = Build Array(0.0 ("Element"), 0.0 ("Element"), 0.0 ("Element")) -> (w554:dbl[])
        n218 = while {
          tunnel: w543 -> [w622]
          tunnel: w536 -> [w602]
          shift-right: [w574] -> _
          shift-left: w537 -> [w617]
          shift-right: [w591] -> _
          shift-left: dbl[][] [] -> [w592]
          shift-right: [w593] -> _
          shift-left: string[] ["Time, Event mark"] -> [w594]
          tunnel: w510 -> [w564]
          i -> [w573]
          stop <- w618 stop-if-true
          # "Replace time axis"
          # "Calculate average values"
          # "Determine dV"
          # "Combine traces for regression"
          n219 = local read "Stop recording"() -> (w619:bool)
          n220 = Dequeue Element(queue=w622) -> (element=w597:cluster{string[], dbl[][]}, error out=w621:errorcluster)  [unwired: 2 in, 2 out]
          n221 = local read "Start fit (% of rec. period)"() -> (w606:dbl)
          n222 = Greater Or Equal?(x=w573, y=2) -> (x >= y?=w584:bool)
          n223 = Unbundle By Name(w621) -> ("status"=w620:bool)
          n224 = Or(x=w620, y=w619) -> (x .or. y?=w618:bool)
          n225 = Unbundle(w597) -> (w595:string[], w596:dbl[][])
          n226 = Multiply(x=w602, y=w606) -> (x*y=w587:dbl)
          n227 = Multiply(x=w602, y=100.0) -> (x*y=w588:dbl)
          n228 = Multiply(x=w602, y=100.0) -> (x*y=w615:dbl)
          n229 = Multiply(x=w602, y=200.0) -> (x*y=w614:dbl)
          n230 = Array Subset(array=w617, index (row)=w615, length (row)=w614) -> (w611:dbl[][])  [unwired: 2 in]
          n231 = Delete From Array(array=w596, index (col)=1 ("Deaktivierter Index (Spalte)")) -> (array with subset deleted=w610:dbl[][])  [unwired: 2 in, 1 out]
          n232 = Insert Into Array(array=w611, new element=w610) -> (w574:dbl[][])  [unwired: 2 in]
          n233 = local read "Start fit (% of rec. period)"() -> (w603:dbl)
          n234 = Multiply(x=w602, y=w603) -> (x*y=w600:dbl)
          n235 = Multiply(x=w602, y=100.0) -> (x*y=w599:dbl)
          n236 = Add(x=w600, y=w599) -> (x+y=w601:dbl)
          n237 = Subtract(x=w599, y=w600) -> (x-y=w589:dbl)
          n238 = Array Subset(array=w574, index (row)=w601, length (row)=w589) -> (w576:dbl[][])  [unwired: 2 in]
          n239 = Transpose 2D Array(2D array=w576) -> (transposed array=w575:dbl[][])
          n240 = for {
            tunnel: w575 -> [w711] mode=indexing
            shift-right: [w710] -> w579
            shift-left: dbl[] [] -> [w709]
            n241 = Add Array Elements(numeric array=w711) -> (sum=w712:dbl)
            n242 = Array Size(array=w711) -> (size(s)=w713:i32)
            n243 = Divide(x=w712, y=w713) -> (x/y=w708:dbl)
            n244 = Insert Into Array(array=w709, new element=w708) -> (w710:dbl[])  [unwired: 1 in]
          }
          n245 = Index Array(array=w574, index (col)=0 ("Deaktivierter Index (Spalte)")) -> (element=w583:dbl[])  [unwired: 1 in]
          n246 = Index Array(array=w579, index=0 ("Index (Spalte)")) -> (element=w581:dbl)
          n247 = for {
            tunnel: w581 -> [w1052]
            shift-right: [w1055] -> w607
            shift-left: dbl[] [] -> [w1054]
            tunnel: w583 -> [w1051] mode=indexing
            n248 = Subtract(x=w1051, y=w1052) -> (x-y=w1053:dbl)
            n249 = Insert Into Array(array=w1054, new element=w1053) -> (w1055:dbl[])  [unwired: 1 in]
          }
          n250 = Replace Array Subset(array=w574, new element=w607, index (col)=0 ("Deaktivierter Index (Spalte)")) -> (w580:dbl[][])  [unwired: 1 in]
          n251 = for {
            N: 2 -> [_]
            tunnel: w580 -> [w638]
            tunnel: w588 -> [w637]
            tunnel: w587 -> [w636]
            tunnel: w584 -> [w632]
            tunnel: w573 -> [w630]
            shift-right: [w629] -> w577
            shift-left: dbl[] [] -> [w628]
            i -> [w635]
            n252 = flat-sequence {
              tunnel: w638 -> [w649]
              tunnel: w636 -> [w650]
              tunnel: w637 -> [w657]
              tunnel: [w654] -> w640
              tunnel: [w651] -> w639
              tunnel: w631 -> [w645]
              tunnel: w640 -> [w681]
              tunnel: w639 -> [w687]
              tunnel: w630 -> [w682]
              tunnel: [w670] -> w627
              tunnel: [w669] -> w633
              frame #0 {
                n253 = Subtract(x=w657, y=w650) -> (x-y=w663:dbl)
                n254 = Multiply(x=w657, y=2.0) -> (x*y=w660:dbl)
                n255 = Add(x=w650, y=w660) -> (x+y=w668:dbl)
                n256 = Add(x=w650, y=w657) -> (x+y=w667:dbl)
                n257 = Array Subset(array=w649, index (row)=w650, length (row)=w663) -> (w665:dbl[][])  [unwired: 2 in]
                n258 = Array Subset(array=w649, index (row)=w668, length (row)=w663) -> (w666:dbl[][])  [unwired: 2 in]
                n259 = Array Subset(array=w649, index (row)=w667, length (row)=w663) -> (w658:dbl[][])  [unwired: 2 in]
                n260 = Insert Into Array(array=w665, new element=w666) -> (w661:dbl[][])  [unwired: 2 in]
                n261 = Index Array(array=w658, index (col)=w645) -> (element=w648:dbl[])  [unwired: 1 in]
                n262 = Index Array(array=w661, index (col)=0 ("disabled index (col)")) -> (element=w656:dbl[])  [unwired: 1 in]
                n263 = Index Array(array=w658, index (col)=0 ("disabled index (col)")) -> (element=w647:dbl[])  [unwired: 1 in]
                n264 = Index Array(array=w661, index (col)=w645) -> (element=w655:dbl[])  [unwired: 1 in]
                n265 = call <vilib>:"Linear Fit.vi"("Y"=w655, "X"=w656) -> ("Best Linear Fit"=w646:dbl[], "slope"=w653:dbl, "intercept"=w652:dbl)  [unwired: 9 in, 2 out]
                n266 = Build Array(w653, w652) -> (w651:dbl[])
                n267 = Bundle(w656, w655, "Best Linear Fit"=w646, w647, w648) -> (w654:T8)  [unwired: 1 in]
              }
              frame #1 {
                n268 = Unbundle(w681) -> (w692:dbl[], w693:dbl[])  [unwired: 3 out]
                n269 = Divide(x=w682, y=2 ("x")) -> (x/y=w683:dbl)
                n270 = Index Array(array=w687, index=0 ("Index")) -> (element=w694:dbl)
                n271 = Index Array(array=w687, index=1 ("Index")) -> (element=w686:dbl)
                n272 = Unbundle(w681) -> (w678:dbl[], w680:dbl[], "Best Linear Fit"=w677:dbl[], w676:dbl[], w674:dbl[])
                n273 = Round To Nearest(number=w683) -> (nearest integer value=w684:dbl)
                n274 = Absolute Value(x=w694) -> (abs(x)=w699:dbl)
                n275 = Equal?(x=w684, y=w683) -> (x = y?=w689:bool)
                n276 = Divide(x=w699, y=1000.0) -> (x/y=w701:dbl)
                n277 = Bundle(w678, w680) -> (w679:cluster{dbl[], dbl[]})  [unwired: 1 in]
                n278 = Bundle(w678, "Best Linear Fit"=w677) -> (w673:cluster{dbl[], "Best Linear Fit":dbl[]})  [unwired: 1 in]
                n279 = Bundle(w676, w674) -> (w671:cluster{dbl[], dbl[]})  [unwired: 1 in]
                n280 = Subtract(x=w694, y=w701) -> (x-y=w698:dbl)
                n281 = Add(x=w694, y=w701) -> (x+y=w697:dbl)
                n282 = Bundle(w698, w697, -inf, inf) -> (w696:cluster{dbl, dbl, dbl, dbl})  [unwired: 1 in]
                n283 = call <vilib>:"Linear Fit.vi"("Y"=w693, "X"=w692, "parameter bounds"=w696) -> ("Best Linear Fit"=w675:dbl[], "intercept"=w685:dbl)  [unwired: 8 in, 3 out]
                n284 = Subtract(x=w686, y=w685) -> (x-y=w690:dbl)
                n285 = Bundle(w676, "Best Linear Fit"=w675) -> (w672:cluster{dbl[], "Best Linear Fit":dbl[]})  [unwired: 1 in]
                n286 = case shown="True" w689 {
                  tunnel: w690 -> [w704 w706]
                  tunnel: [w704 w707] -> w670
                  frame False {
                  }
                  frame True {
                    n287 = Multiply(x=-1.0, y=w706) -> (x*y=w707:dbl)
                  }
                }
                n288 = Build Array(w679, w673, w672, w671) -> (w669:cluster{dbl[], "Best Linear Fit":dbl[]}[])
              }
            }
            n289 = Add(x=1, y=w635) -> (x+y=w631:i32)
            n290 = case shown="True" w632 {
              tunnel: w633 -> [_ w642]
              tunnel: w631 -> [_ w641]
              frame False {
              }
              frame True {
                n291 = case shown="0, Default" w641 {
                  tunnel: w642 -> [_ w643 w644]
                  frame 0, Default {
                  }
                  frame 1 {
                    "deltaV SISE 1" <- w643
                  }
                  frame 2 {
                    "deltaV SISE 2" <- w644
                  }
                }
              }
            }
            n292 = Insert Into Array(array=w628, new element=w627) -> (w629:dbl[])  [unwired: 1 in]
          }
          n293 = Insert Into Array(array=w579, index=3 ("Index"), new element=w577) -> (w566:dbl[])
          n294 = Index Array(array=w566, index=0 ("Index")) -> (element=w568:dbl)
          n295 = Divide(x=w568, y=60.0) -> (x/y=w567:dbl)
          n296 = Replace Array Subset(array=w566, new element=w567, index=0 ("Index")) -> (w565:dbl[])
          n297 = case shown="True" w584 {
            tunnel: w592 -> [w623 w626]
            tunnel: [w623 w625] -> w591
            tunnel: w565 -> [_ w624]
            frame False {
            }
            frame True {
              n298 = Insert Into Array(array=w626, new element=w624) -> (w625:dbl[][])  [unwired: 2 in]
            }
          }
          n299 = while {
            tunnel: w591 -> [w720]
            tunnel: w595 -> [w737]
            tunnel: w594 -> [w736]
            tunnel: [w727] -> w593
            tunnel: w573 -> [w726]
            tunnel: w573 -> [w721]
            tunnel: w564 -> [w719]
            i -> [w771]
            stop <- w716 stop-if-true
            n300 = for {
              tunnel: w737 -> [w1031] mode=indexing
              shift-right: [w1028] -> w722
              shift-left: TRUE -> [w1032]
              n301 = Equal?(x=w1031, y="") -> (x = y?=w1029:bool)
              n302 = case shown="True" w1029 {
                tunnel: w1032 -> [_ w1034]
                tunnel: [FALSE w1034] -> w1028
                frame False {
                }
                frame True {
                }
              }
            }
            n303 = Wait (ms)(milliseconds to wait=u32 100 ("Zu wartende ms")) -> ()  [unwired: 1 out]
            n304 = Multiply(x="Zoom from end", y=-1.0) -> (x*y=w755:dbl)
            n305 = Add(x="Zoom from start", y=w755) -> (x+y=w766:dbl)
            n306 = feedback #4() -> (w761:dbl)  [unwired: 1 in]
            n307 = Greater Or Equal?(x=w766, y=0.0) -> (x >= y?=w764:bool)
            n308 = Less?(x=w726, y=2) -> (x < y?=w724:bool)
            n309 = case shown="True" w764 {
              tunnel: "Zoom from start" -> [w1043 w1046]
              tunnel: [w1042 w1046] -> w762
              tunnel: w761 -> [w1042 w1048]
              tunnel: "Zoom from end" -> [_ w1045]
              tunnel: [w1043 w1046] -> w754
              tunnel: [w1041 w1044] -> w753
              tunnel: "Zoom from end" -> [w1041 w1044]
              frame False {
              }
              frame True {
                n310 = Not Equal?(x=w1048, y=w1046) -> (x != y?=w1047:bool)
                n311 = case shown="False" w1047 {
                  tunnel: w1046 -> [_ w1050]
                  tunnel: w1045 -> [w1049 _]
                  frame False {
                    n312 = local write "Zoom from start"(w1049) -> ()
                  }
                  frame True {
                    n313 = local write "Zoom from end"(w1050) -> ()
                  }
                }
              }
            }
            n314 = feedback-in #4(w762) -> ()
            n315 = Or(x=w722, y=w724) -> (x .or. y?=w723:bool)
            n316 = case shown="False" w723 {
              tunnel: w736 -> [w1024 w1027]
              tunnel: [w1026 w1027] -> w727
              tunnel: w737 -> [w1025 _]
              frame False {
                n317 = Insert Into Array(array=w1024, new element=w1025) -> (w1026:string[])  [unwired: 1 in]
              }
              frame True {
              }
            }
            n318 = Array Size(array=w727) -> (size(s)=w733:i32)
            n319 = Array Subset(array=w727, index=1 ("Index")) -> (w741:string[])  [unwired: 1 in]
            n320 = Subtract(x=w753, y=w754) -> (x-y=w760:dbl)
            n321 = Divide(x=w733, y=10) -> (x/y=w731:dbl)
            n322 = for {
              tunnel: w741 -> [w1037] mode=indexing
              shift-right: [w1040] -> w739
              shift-left: dbl[] [] -> [w1039]
              n323 = Match Pattern(string=w1037, regular expression="\t") -> (before substring=w1035:string)  [unwired: 1 in, 3 out]
              n324 = Fract/Exp String To Number(string=w1035) -> (number=w1038:dbl)  [unwired: 3 in, 1 out]
              n325 = Insert Into Array(array=w1039, new element=w1038) -> (w1040:dbl[])  [unwired: 1 in]
            }
            n326 = Index Array(array=w720, index (col)=0 ("Deaktivierter Index (Spalte)")) -> (element=w768:dbl[])  [unwired: 1 in]
            n327 = Multiply(x=w731, y="Bildlaufleiste") -> (x*y=w729:dbl)
            n328 = Divide(x=w754, y=100.0) -> (x/y=w756:dbl)
            n329 = Divide(x=w760, y=100.0) -> (x/y=w757:dbl)
            n330 = Array Size(array=w768) -> (size(s)=w750:i32)
            n331 = Array Subset(array=w727, index=w729) -> (w728:string[])  [unwired: 1 in]
            n332 = Multiply(x=w750, y=w756) -> (x*y=w746:dbl)
            n333 = Multiply(x=w750, y=w757) -> (x*y=w749:dbl)
            n334 = Index Array(array=w719, index="TC 3") -> (element=w718:bool)
            n335 = Add(x=w749, y=2.0) -> (x+y=w747:dbl)
            n336 = Subtract(x=w746, y=2.0) -> (x-y=w744:dbl)
            n337 = for {
              shift-right: [w1022] -> w734
              shift-left: "" -> [w1023]
              tunnel: w728 -> [w1020] mode=indexing
              n338 = Concatenate Strings(w1023, w1020, "\r") -> (w1022:string)
            }
            "?" <- w734
            n339 = Array Subset(array=w720, index (row)=w744, length (row)=w747) -> (w740:dbl[][])  [unwired: 2 in]
            n340 = case shown="\"V channel #1\"" "TC 3" {
              tunnel: w740 -> [w783 w863 w975 w986]
              tunnel: w739 -> [w781 w862 w943 w989]
              tunnel: w721 -> [w780 w859 w940 w981]
              tunnel: w718 -> [w777 w858 w939 w980]
              frame "SISE channel #1", Default {
                n341 = Greater Or Equal?(x=w780, y=2) -> (x >= y?=w778:bool)
                n342 = And(x=w778, y=w777) -> (x .and. y?=w776:bool)
                n343 = Index Array(array=w783, index (col)=0 ("disabled index (col)")) -> (element=w786:dbl[])  [unwired: 1 in]
                n344 = Index Array(array=w783, index (col)=1 ("disabled index (col)")) -> (element=w785:dbl[])  [unwired: 1 in]
                n345 = Index Array(array=w783, index (col)=3 ("disabled index (col)")) -> (element=w782:dbl[])  [unwired: 1 in]
                n346 = stacked-sequence {
                  tunnel: w786 -> [w790 w829]
                  tunnel: w785 -> [w809 _]
                  tunnel: w781 -> [w791 w828]
                  tunnel: w782 -> [_ w827]
                  tunnel: w776 -> [w789 w823]
                  frame #0 {
                    n347 = Array Max & Min(array=w790) -> (max value=w801:dbl, min value=w800:dbl)  [unwired: 2 out]
                    n348 = Divide(x="Range limit\nS1.1 (mV)", y=2.0) -> (x/y=w819:dbl)
                    n349 = Divide(x="Range limit\nS1.1 (mV)", y=2.05) -> (x/y=w820:dbl)
                    n350 = Add(x="Base line\nS1.1 (mV)", y=w819) -> (x+y=w792:dbl)
                    n351 = Subtract(x="Base line\nS1.1 (mV)", y=w819) -> (x-y=w793:dbl)
                    n352 = Subtract(x="Base line\nS1.1 (mV)", y=w820) -> (x-y=w799:dbl)
                    n353 = call "EventstoGraph (SubVI).vi"("Numerisch 2"=w800, "Array 3"=w791, "Numerisch"=w801, "Array (Eingang)"=dbl[][] [], "Numerisch 3"=w799) -> ("Array (Ausgang)"=w803:dbl[][])  [unwired: 6 in]
                    n354 = Array Max & Min(array=w790) -> (max value=w815:dbl, min value=w816:dbl)  [unwired: 2 out]
                    n355 = call "GraphLimit01.vi"("Numeric 2"=w793, "Numeric"=w792, "Array in"=w809, "Array 3"=dbl[] []) -> ("Array out"=w808:dbl[])  [unwired: 7 in]
                    n356 = Build Array("Base line\nS1.1 (mV)", "Base line\nS1.1 (mV)") -> (w812:dbl[])
                    n357 = Build Array(w815, w816) -> (w813:dbl[])
                    n358 = Build Array(w792, w793) -> (w814:dbl[])
                    n359 = Index Array(array=w803, index (col)=0 ("Index (Zeile)")) -> (element=w804:dbl[])  [unwired: 1 in]
                    n360 = Index Array(array=w803, index (col)=1 ("Index (Zeile)")) -> (element=w802:dbl[])  [unwired: 1 in]
                    n361 = Bundle(w813, w814) -> (w796:cluster{dbl[], dbl[]})  [unwired: 1 in]
                    n362 = Bundle(w813, w812) -> (w797:cluster{dbl[], dbl[]})  [unwired: 1 in]
                    n363 = Bundle(w790, "Array out"=w808) -> (w795:cluster{dbl[], "Array out":dbl[]})  [unwired: 1 in]
                    n364 = Bundle("Array (Ausgang)"=w804, "Array (Ausgang)"=w802) -> (w794:T9)  [unwired: 1 in]
                    n365 = Build Array(w797, w796, w795, w794) -> (w798:T10)
                    n366 = case shown="True" w789 {
                      tunnel: w798 -> [_ w822]
                      frame False {
                      }
                      frame True {
                        "V-SISE channel 1" <- w822
                      }
                    }
                  }
                  frame #1 {
                    n367 = Array Max & Min(array=w829) -> (max value=w838:dbl, min value=w837:dbl)  [unwired: 2 out]
                    n368 = Divide(x="Range limit\nS1.2 mV", y=2.0) -> (x/y=w854:dbl)
                    n369 = Divide(x="Range limit\nS1.2 mV", y=2.05) -> (x/y=w855:dbl)
                    n370 = Add(x="Base line \nS1.2 (mV)", y=w854) -> (x+y=w830:dbl)
                    n371 = Subtract(x="Base line \nS1.2 (mV)", y=w854) -> (x-y=w831:dbl)
                    n372 = Subtract(x="Base line \nS1.2 (mV)", y=w855) -> (x-y=w836:dbl)
                    n373 = call "EventstoGraph (SubVI).vi"("Numerisch 2"=w837, "Array 3"=w828, "Numerisch"=w838, "Array (Eingang)"=dbl[][] [], "Numerisch 3"=w836) -> ("Array (Ausgang)"=w840:dbl[][])  [unwired: 6 in]
                    n374 = Array Max & Min(array=w829) -> (max value=w850:dbl, min value=w851:dbl)  [unwired: 2 out]
                    n375 = call "GraphLimit01.vi"("Numeric 2"=w831, "Numeric"=w830, "Array in"=w827, "Array 3"=dbl[] []) -> ("Array out"=w845:dbl[])  [unwired: 7 in]
                    n376 = Build Array("Base line \nS1.2 (mV)", "Base line \nS1.2 (mV)") -> (w847:dbl[])
                    n377 = Build Array(w850, w851) -> (w848:dbl[])
                    n378 = Build Array(w830, w831) -> (w849:dbl[])
                    n379 = Index Array(array=w840, index (col)=0 ("Index (Zeile)")) -> (element=w841:dbl[])  [unwired: 1 in]
                    n380 = Index Array(array=w840, index (col)=1 ("Index (Zeile)")) -> (element=w839:dbl[])  [unwired: 1 in]
                    n381 = Bundle(w848, w849) -> (w834:cluster{dbl[], dbl[]})  [unwired: 1 in]
                    n382 = Bundle(w848, w847) -> (w835:cluster{dbl[], dbl[]})  [unwired: 1 in]
                    n383 = Bundle(w829, "Array out"=w845) -> (w833:cluster{dbl[], "Array out":dbl[]})  [unwired: 1 in]
                    n384 = Bundle("Array (Ausgang)"=w841, "Array (Ausgang)"=w839) -> (w832:T9)  [unwired: 1 in]
                    n385 = Build Array(w835, w834, w833, w832) -> (w824:T10)
                    n386 = case shown="True" w823 {
                      tunnel: w824 -> [_ w856]
                      frame False {
                      }
                      frame True {
                        "dV-SISE channel 1" <- w856
                      }
                    }
                  }
                }
              }
              frame "SISE channel #2" {
                n387 = Greater Or Equal?(x=w859, y=2) -> (x >= y?=w861:bool)
                n388 = And(x=w861, y=w858) -> (x .and. y?=w857:bool)
                n389 = Index Array(array=w863, index (col)=0 ("disabled index (col)")) -> (element=w867:dbl[])  [unwired: 1 in]
                n390 = Index Array(array=w863, index (col)=2 ("disabled index (col)")) -> (element=w868:dbl[])  [unwired: 1 in]
                n391 = Index Array(array=w863, index (col)=4 ("disabled index (col)")) -> (element=w869:dbl[])  [unwired: 1 in]
                n392 = stacked-sequence {
                  tunnel: w867 -> [w871 w910]
                  tunnel: w868 -> [w890 _]
                  tunnel: w862 -> [w872 w909]
                  tunnel: w869 -> [_ w908]
                  tunnel: w857 -> [w870 w904]
                  frame #0 {
                    n393 = Array Max & Min(array=w871) -> (max value=w882:dbl, min value=w881:dbl)  [unwired: 2 out]
                    n394 = Divide(x="Range limit\nS2.1 (mV)", y=2.0) -> (x/y=w900:dbl)
                    n395 = Divide(x="Range limit\nS2.1 (mV)", y=2.05) -> (x/y=w901:dbl)
                    n396 = Add(x="Base line\nS2.1 (mV)", y=w900) -> (x+y=w873:dbl)
                    n397 = Subtract(x="Base line\nS2.1 (mV)", y=w900) -> (x-y=w874:dbl)
                    n398 = Subtract(x="Base line\nS2.1 (mV)", y=w901) -> (x-y=w880:dbl)
                    n399 = call "EventstoGraph (SubVI).vi"("Numerisch 2"=w881, "Array 3"=w872, "Numerisch"=w882, "Array (Eingang)"=dbl[][] [], "Numerisch 3"=w880) -> ("Array (Ausgang)"=w884:dbl[][])  [unwired: 6 in]
                    n400 = Array Max & Min(array=w871) -> (max value=w896:dbl, min value=w897:dbl)  [unwired: 2 out]
                    n401 = call "GraphLimit01.vi"("Numeric 2"=w874, "Numeric"=w873, "Array in"=w890, "Array 3"=dbl[] []) -> ("Array out"=w889:dbl[])  [unwired: 7 in]
                    n402 = Build Array("Base line\nS2.1 (mV)", "Base line\nS2.1 (mV)") -> (w893:dbl[])
                    n403 = Build Array(w896, w897) -> (w894:dbl[])
                    n404 = Build Array(w873, w874) -> (w895:dbl[])
                    n405 = Index Array(array=w884, index (col)=0 ("Index (Zeile)")) -> (element=w885:dbl[])  [unwired: 1 in]
                    n406 = Index Array(array=w884, index (col)=1 ("Index (Zeile)")) -> (element=w883:dbl[])  [unwired: 1 in]
                    n407 = Bundle(w894, w895) -> (w877:cluster{dbl[], dbl[]})  [unwired: 1 in]
                    n408 = Bundle(w894, w893) -> (w878:cluster{dbl[], dbl[]})  [unwired: 1 in]
                    n409 = Bundle(w871, "Array out"=w889) -> (w876:cluster{dbl[], "Array out":dbl[]})  [unwired: 1 in]
                    n410 = Bundle("Array (Ausgang)"=w885, "Array (Ausgang)"=w883) -> (w875:T9)  [unwired: 1 in]
                    n411 = Build Array(w878, w877, w876, w875) -> (w879:T10)
                    n412 = case shown="True" w870 {
                      tunnel: w879 -> [_ w903]
                      frame False {
                      }
                      frame True {
                        "V-SISE channel 2" <- w903
                      }
                    }
                  }
                  frame #1 {
                    n413 = Array Max & Min(array=w910) -> (max value=w919:dbl, min value=w918:dbl)  [unwired: 2 out]
                    n414 = Divide(x="Range limit\nS2.2 (mV)", y=2.0) -> (x/y=w935:dbl)
                    n415 = Divide(x="Range limit\nS2.2 (mV)", y=2.05) -> (x/y=w936:dbl)
                    n416 = Add(x="Base line \nS2.2 (mV)", y=w935) -> (x+y=w911:dbl)
                    n417 = Subtract(x="Base line \nS2.2 (mV)", y=w935) -> (x-y=w912:dbl)
                    n418 = Subtract(x="Base line \nS2.2 (mV)", y=w936) -> (x-y=w917:dbl)
                    n419 = call "EventstoGraph (SubVI).vi"("Numerisch 2"=w918, "Array 3"=w909, "Numerisch"=w919, "Array (Eingang)"=dbl[][] [], "Numerisch 3"=w917) -> ("Array (Ausgang)"=w921:dbl[][])  [unwired: 6 in]
                    n420 = Array Max & Min(array=w910) -> (max value=w931:dbl, min value=w932:dbl)  [unwired: 2 out]
                    n421 = call "GraphLimit01.vi"("Numeric 2"=w912, "Numeric"=w911, "Array in"=w908, "Array 3"=dbl[] []) -> ("Array out"=w926:dbl[])  [unwired: 7 in]
                    n422 = Build Array("Base line \nS2.2 (mV)", "Base line \nS2.2 (mV)") -> (w928:dbl[])
                    n423 = Build Array(w931, w932) -> (w929:dbl[])
                    n424 = Build Array(w911, w912) -> (w930:dbl[])
                    n425 = Index Array(array=w921, index (col)=0 ("Index (Zeile)")) -> (element=w922:dbl[])  [unwired: 1 in]
                    n426 = Index Array(array=w921, index (col)=1 ("Index (Zeile)")) -> (element=w920:dbl[])  [unwired: 1 in]
                    n427 = Bundle(w929, w930) -> (w915:cluster{dbl[], dbl[]})  [unwired: 1 in]
                    n428 = Bundle(w929, w928) -> (w916:cluster{dbl[], dbl[]})  [unwired: 1 in]
                    n429 = Bundle(w910, "Array out"=w926) -> (w914:cluster{dbl[], "Array out":dbl[]})  [unwired: 1 in]
                    n430 = Bundle("Array (Ausgang)"=w922, "Array (Ausgang)"=w920) -> (w913:T9)  [unwired: 1 in]
                    n431 = Build Array(w916, w915, w914, w913) -> (w905:T10)
                    n432 = case shown="True" w904 {
                      tunnel: w905 -> [_ w937]
                      frame False {
                      }
                      frame True {
                        "dV-SISE channel 2" <- w937
                      }
                    }
                  }
                }
              }
              frame "V channel #1" {
                n433 = Greater Or Equal?(x=w940, y=2) -> (x >= y?=w942:bool)
                n434 = And(x=w942, y=w939) -> (x .and. y?=w938:bool)
                n435 = Index Array(array=w975, index (col)=0 ("disabled index (col)")) -> (element=w944:dbl[])  [unwired: 1 in]
                n436 = Index Array(array=w975, index (col)=5 ("disabled index (col)")) -> (element=w945:dbl[])  [unwired: 1 in]
                n437 = Array Max & Min(array=w944) -> (max value=w955:dbl, min value=w954:dbl)  [unwired: 2 out]
                n438 = Divide(x="Range limit\nV1 (V)", y=2.0) -> (x/y=w972:dbl)
                n439 = Divide(x="Range limit\nV1 (V)", y=2.05) -> (x/y=w973:dbl)
                n440 = Add(x="Base line\nV1 (V)", y=w972) -> (x+y=w946:dbl)
                n441 = Subtract(x="Base line\nV1 (V)", y=w972) -> (x-y=w947:dbl)
                n442 = Subtract(x="Base line\nV1 (V)", y=w973) -> (x-y=w953:dbl)
                n443 = call "EventstoGraph (SubVI).vi"("Numerisch 2"=w954, "Array 3"=w943, "Numerisch"=w955, "Array (Eingang)"=dbl[][] [], "Numerisch 3"=w953) -> ("Array (Ausgang)"=w957:dbl[][])  [unwired: 6 in]
                n444 = Array Max & Min(array=w944) -> (max value=w968:dbl, min value=w969:dbl)  [unwired: 2 out]
                n445 = call "GraphLimit01.vi"("Numeric 2"=w947, "Numeric"=w946, "Array in"=w945, "Array 3"=dbl[] []) -> ("Array out"=w962:dbl[])  [unwired: 7 in]
                n446 = Build Array("Base line\nV1 (V)", "Base line\nV1 (V)") -> (w965:dbl[])
                n447 = Build Array(w968, w969) -> (w966:dbl[])
                n448 = Build Array(w946, w947) -> (w967:dbl[])
                n449 = Index Array(array=w957, index (col)=0 ("Index (Zeile)")) -> (element=w958:dbl[])  [unwired: 1 in]
                n450 = Index Array(array=w957, index (col)=1 ("Index (Zeile)")) -> (element=w956:dbl[])  [unwired: 1 in]
                n451 = Bundle(w966, w967) -> (w950:cluster{dbl[], dbl[]})  [unwired: 1 in]
                n452 = Bundle(w966, w965) -> (w951:cluster{dbl[], dbl[]})  [unwired: 1 in]
                n453 = Bundle(w944, "Array out"=w962) -> (w949:cluster{dbl[], "Array out":dbl[]})  [unwired: 1 in]
                n454 = Bundle("Array (Ausgang)"=w958, "Array (Ausgang)"=w956) -> (w948:T9)  [unwired: 1 in]
                n455 = Build Array(w951, w950, w949, w948) -> (w952:T10)
                n456 = case shown="True" w938 {
                  tunnel: w952 -> [_ w978]
                  frame False {
                  }
                  frame True {
                    "Voltage channel 1" <- w978
                  }
                }
              }
              frame "V channel #2" {
                n457 = Greater Or Equal?(x=w981, y=2) -> (x >= y?=w982:bool)
                n458 = And(x=w982, y=w980) -> (x .and. y?=w979:bool)
                n459 = Index Array(array=w986, index (col)=0 ("disabled index (col)")) -> (element=w984:dbl[])  [unwired: 1 in]
                n460 = Index Array(array=w986, index (col)=6 ("disabled index (col)")) -> (element=w985:dbl[])  [unwired: 1 in]
                n461 = Array Max & Min(array=w984) -> (max value=w999:dbl, min value=w998:dbl)  [unwired: 2 out]
                n462 = Divide(x="Range limit\nV2 (V)", y=2.0) -> (x/y=w1016:dbl)
                n463 = Divide(x="Range limit\nV2 (V)", y=2.05) -> (x/y=w1017:dbl)
                n464 = Add(x="Base line\nV2 (V)", y=w1016) -> (x+y=w990:dbl)
                n465 = Subtract(x="Base line\nV2 (V)", y=w1016) -> (x-y=w991:dbl)
                n466 = Subtract(x="Base line\nV2 (V)", y=w1017) -> (x-y=w997:dbl)
                n467 = call "EventstoGraph (SubVI).vi"("Numerisch 2"=w998, "Array 3"=w989, "Numerisch"=w999, "Array (Eingang)"=dbl[][] [], "Numerisch 3"=w997) -> ("Array (Ausgang)"=w1001:dbl[][])  [unwired: 6 in]
                n468 = Array Max & Min(array=w984) -> (max value=w1012:dbl, min value=w1013:dbl)  [unwired: 2 out]
                n469 = call "GraphLimit01.vi"("Numeric 2"=w991, "Numeric"=w990, "Array in"=w985, "Array 3"=dbl[] []) -> ("Array out"=w1006:dbl[])  [unwired: 7 in]
                n470 = Build Array("Base line\nV2 (V)", "Base line\nV2 (V)") -> (w1009:dbl[])
                n471 = Build Array(w1012, w1013) -> (w1010:dbl[])
                n472 = Build Array(w990, w991) -> (w1011:dbl[])
                n473 = Index Array(array=w1001, index (col)=0 ("Index (Zeile)")) -> (element=w1002:dbl[])  [unwired: 1 in]
                n474 = Index Array(array=w1001, index (col)=1 ("Index (Zeile)")) -> (element=w1000:dbl[])  [unwired: 1 in]
                n475 = Bundle(w1010, w1011) -> (w994:cluster{dbl[], dbl[]})  [unwired: 1 in]
                n476 = Bundle(w1010, w1009) -> (w995:cluster{dbl[], dbl[]})  [unwired: 1 in]
                n477 = Bundle(w984, "Array out"=w1006) -> (w993:cluster{dbl[], "Array out":dbl[]})  [unwired: 1 in]
                n478 = Bundle("Array (Ausgang)"=w1002, "Array (Ausgang)"=w1000) -> (w992:T9)  [unwired: 1 in]
                n479 = Build Array(w995, w994, w993, w992) -> (w996:T10)
                n480 = case shown="True" w979 {
                  tunnel: w996 -> [_ w1019]
                  frame False {
                  }
                  frame True {
                    "Voltage channel 2" <- w1019
                  }
                }
              }
            }
            n481 = local read "Record period (round at 5s)"() -> (w770:dbl)
            n482 = local read "Stop recording 2"() -> (w714:bool)
            n483 = Multiply(x=w770, y=10.0) -> (x*y=w774:dbl)
            n484 = Subtract(x=w774, y=10.0) -> (x-y=w772:dbl)
            n485 = Greater Or Equal?(x=w771, y=w772) -> (x >= y?=w715:bool)
            n486 = Or(x=w714, y=w715) -> (x .or. y?=w716:bool)
          }
        }
        n487 = while {
          tunnel: w540 -> [w1083]
          tunnel: w559 -> [w1101]
          tunnel: w553 -> [w1094]
          shift-right: [w1093] -> _
          shift-left: "P0: P1:" -> [w1096]
          shift-right: [w1092] -> _
          shift-left: w554 -> [w1095]
          tunnel: [w1091] -> w552
          tunnel: w551 -> [w1090]
          tunnel: [w1085] -> w514
          tunnel: [w1084] -> w513
          shift-right: [w1078] -> w545
          shift-left: w543 -> [w1076]
          shift-right: [w1077] -> w544
          shift-left: w546 -> [w1081]
          tunnel: w530 -> [w1073]
          tunnel: [w1067] -> w512
          tunnel: [w1066] -> w511
          shift-right: [w1062] -> _
          shift-left: "" -> [w1064]
          tunnel: string[] [] -> [w1065]
          tunnel: [w1063] -> _
          tunnel: w510 -> [w1059]
          tunnel: [w1058] -> w523
          tunnel: w510 -> [w1056]
          i -> [w1061]
          stop <- w1057 stop-if-true
          n488 = Unbundle(w1090) -> ("task out"=w1060:refnum<k21>, "status"=w1089:bool, "code"=w1088:i32, "source"=w1087:string)
          n489 = Unbundle(w1073) -> ("refnum out"=w1069:refnum<file>, "status"=w1072:bool, "code"=w1070:i32, "source"=w1071:string)
          n490 = Divide(x=w1061, y=2) -> (x/y=w1099:dbl)
          n491 = Round Toward -Infinity(1:w1099) -> (0:w1100:dbl)
          n492 = Bundle("status"=w1089, "code"=w1088, "source"=w1087) -> (w1086:errorcluster)  [unwired: 1 in]
          n493 = Bundle("status"=w1072, "code"=w1070, "source"=w1071) -> (w1068:errorcluster)  [unwired: 1 in]
          n494 = Equal?(x=w1099, y=w1100) -> (x = y?=w1097:bool)
          n495 = while {
            tunnel: w1083 -> [w1221]
            shift-right: [w1121] -> w1057
            shift-left: FALSE -> [w1217]
            tunnel: w1101 -> [w1215]
            tunnel: w1097 -> [w1138]
            tunnel: w1061 -> [w1205]
            tunnel: w1083 -> [w1158]
            tunnel: w1083 -> [w1198]
            tunnel: w1094 -> [w1197]
            shift-right: [w1122] -> w1093
            shift-left: w1096 -> [w1200]
            shift-right: [w1196] -> w1092
            shift-left: w1095 -> [w1199]
            tunnel: [w1194] -> w1091
            tunnel: w1061 -> [w1186]
            tunnel: w1086 -> [w1184]
            tunnel: w1060 -> [w1185]
            tunnel: [w1144] -> w1085
            tunnel: [w1183] -> w1084
            tunnel: w1083 -> [w1143]
            shift-right: [w1141] -> w1075
            shift-left: dbl[][] [] -> [w1135]
            tunnel: [w1174] -> w1080
            tunnel: [w1173] -> w1079
            tunnel: w1076 -> [w1174]
            tunnel: w1081 -> [w1173]
            tunnel: w1061 -> [w1171]
            tunnel: w1069 -> [w1165]
            tunnel: w1068 -> [w1166]
            tunnel: [w1164] -> w1066
            tunnel: [w1163] -> w1067
            shift-right: [w1160] -> w1063
            shift-left: w1065 -> [w1168]
            shift-right: [w1159] -> w1062
            shift-left: w1064 -> [w1176]
            tunnel: w1061 -> [w1157]
            tunnel: w1059 -> [w1133]
            tunnel: w1059 -> [w1139]
            tunnel: [w1133] -> w1058
            tunnel: w1056 -> [w1105]
            i -> [w1137]
            stop <- w1219 stop-if-true
            w1108 = 0 ("Index")
            # "Write to file"
            # "Add position / Event marks"
            # "Feed graphs"
            # "Get voltage data"
            # "Get time (s) / calculate position of probe"
            # "Control manipulator"
            # "Set graphs and controls"
            # "Set # of cycles"
            # "Stop measurement"
            n496 = Equal?(x=w1157, y=0) -> (x = y?=w1154:bool)
            n497 = Equal?(x=w1137, y=0) -> (x = y?=w1153:bool)
            n498 = Equal To 0?(x=w1137) -> (x = 0?=w1177:bool)
            n499 = Greater Or Equal?(x=w1171, y=2) -> (x >= y?=w1170:bool)
            "E-mark on" <- w1170
            n500 = Get Date/Time In Seconds() -> (seconds since 1Jan1904=w1216:timestamp)
            n501 = call-poly <vilib>:"DAQmx Read.vi"("task/channels in"=w1185, "error in"=w1184) -> ("task out"=w1144:refnum<k21>, "data"=w1107:dbl[][], "error out"=w1183:errorcluster)  [unwired: 11 in]
            n502 = And(x=w1154, y=w1153) -> (x .and. y?=w1152:bool)
            n503 = Index Array(array=w1158, index=2) -> (element=w1203:dbl)
            n504 = Subtract(x=w1216, y=w1215) -> (x-y=w1175:dbl)
            n505 = Multiply(x=w1203, y=100.0) -> (x*y=w1202:dbl)
            n506 = Wait (ms)(milliseconds to wait=u32 10 ("Zu wartende ms")) -> ()  [unwired: 1 out]
            n507 = Index Array(array=w1221, index=2) -> (element=w1224:dbl)
            n508 = case shown="True" w1170 {
              tunnel: [FALSE "Add Mark"] -> w1169
              tunnel: w1168 -> [_ w1290]
              frame False {
              }
              frame True {
                n509 = Array Size(array=w1290) -> (size(s)=w1294:i32)
                n510 = Subtract(x=w1294, y=1) -> (x-y=w1292:i32)
                n511 = Index Array(array=w1290, index=w1292) -> (element=→"String":string)
              }
            }
            n512 = Index Array(array=w1107, index (row)=w1108, index (col)=w1108) -> (element=w1116:dbl)
            n513 = Index Array(array=w1107, index (row)=1 ("Index"), index (col)=w1108) -> (element=w1115:dbl)
            n514 = Index Array(array=w1107, index (row)=2 ("Index"), index (col)=w1108) -> (element=w1113:dbl)
            n515 = Index Array(array=w1107, index (row)=3 ("Index"), index (col)=w1108) -> (element=w1114:dbl)
            n516 = case shown="True" w1152 {
              frame False {
              }
              frame True {
                n517 = Build Array(0.0, 0.0) -> (w1283:dbl[])
                n518 = Build Array(0.0, 30.0) -> (w1284:dbl[])
                n519 = Bundle(w1284, w1283) -> (w1282:cluster{dbl[], dbl[]})  [unwired: 1 in]
                n520 = Build Array(w1282, w1282, w1282, w1282) -> (w1280:cluster{dbl[], dbl[]}[])
                n521 = local write "dV-SISE channel 1"(w1280) -> ()
                n522 = local write "deltaV SISE 1"(w1280) -> ()
                n523 = local write "deltaV SISE 2"(w1280) -> ()
                n524 = local write "V-SISE channel 1"(w1280) -> ()
                n525 = local write "V-SISE channel 2"(w1280) -> ()
                n526 = local write "dV-SISE channel 2"(w1280) -> ()
                n527 = local write "Voltage channel 1"(w1280) -> ()
                n528 = local write "Voltage channel 2"(w1280) -> ()
                n529 = local write "Enable change position 0"(FALSE) -> ()
              }
            }
            n530 = call "Feed-Position-Graph (SubVI).vi"("Array 2"=w1143, "Array"=w1135) -> ("Array 3"=→"Position probe":cluster{dbl[], dbl[]}[])  [unwired: 9 in]
            n531 = Subtract(x=w1202, y=10.0) -> (x-y=w1212:dbl)
            n532 = Subtract(x=w1202, y=20.0) -> (x-y=w1211:dbl)
            n533 = Multiply(x=w1224, y=100.0) -> (x*y=w1208:dbl)
            n534 = Build Array(0, 10, w1211, w1212) -> (w1195:dbl[])
            n535 = Divide(x=w1116, y=-0.0333) -> (x/y=w1111:dbl)
            n536 = Divide(x=w1115, y=-0.0333) -> (x/y=w1112:dbl)
            n537 = Equal?(x=w1205, y=0) -> (x = y?=w1128:bool)
            n538 = Add(x=1 ("y"), y=w1137) -> (x+y=w1220:i32)
            n539 = case shown="False" w1128 {
              tunnel: [w1393 w1411] -> w1127
              tunnel: w1195 -> [w1392 w1410]
              tunnel: w1137 -> [w1391 w1409]
              frame False {
                n540 = for {
                  tunnel: w1392 -> [w1400] mode=indexing
                  tunnel: w1391 -> [w1401]
                  shift-right: [w1398] -> w1393
                  shift-left: 0 -> [w1399]
                  i -> [w1396]
                  n541 = Equal?(x=w1400, y=w1401) -> (x = y?=w1397:bool)
                  n542 = case shown="True" w1397 {
                    tunnel: w1396 -> [_ w1404]
                    tunnel: [0 w1403] -> w1395
                    frame False {
                    }
                    frame True {
                      n543 = case shown="3" w1404 {
                        tunnel: [1 2 3 5] -> w1403
                        frame 0, Default {
                        }
                        frame 1 {
                        }
                        frame 2 {
                        }
                        frame 3 {
                        }
                      }
                    }
                  }
                  n544 = Add(x=w1399, y=w1395) -> (x+y=w1398:i32)
                }
              }
              frame True {
                n545 = for {
                  tunnel: w1410 -> [w1418] mode=indexing
                  tunnel: w1409 -> [w1419]
                  shift-right: [w1416] -> w1411
                  shift-left: 0 -> [w1417]
                  i -> [w1415]
                  n546 = Equal?(x=w1418, y=w1419) -> (x = y?=w1413:bool)
                  n547 = case shown="True" w1413 {
                    tunnel: w1415 -> [_ w1421]
                    tunnel: [0 w1422] -> w1414
                    frame False {
                    }
                    frame True {
                      n548 = case shown="3" w1421 {
                        tunnel: [0 0 3 4] -> w1422
                        frame 0, Default {
                        }
                        frame 1 {
                        }
                        frame 2 {
                        }
                        frame 3 {
                        }
                      }
                    }
                  }
                  n549 = Add(x=w1417, y=w1414) -> (x+y=w1416:i32)
                }
              }
            }
            n550 = Build Array(w1111, w1112, w1113, w1114) -> (w1110:dbl[])
            n551 = Equal?(x=w1208, y=w1220) -> (x = y?=w1219:bool)
            n552 = Index Array(array=w1105, index=4) -> (element=w1103:bool)
            n553 = case shown="True" w1103 {
              tunnel: [-10.0 10.0] -> w1106
              frame False {
              }
              frame True {
              }
            }
            n554 = for {
              tunnel: w1110 -> [w1267] mode=indexing
              tunnel: w1133 -> [w1270] mode=indexing
              shift-right: [w1268] -> w1132
              shift-left: dbl[] [] -> [w1269]
              shift-right: [w1265] -> w1124
              shift-left: dbl[] [] -> [w1266]
              n555 = case shown="False" w1270 {
                tunnel: w1269 -> [w1274 w1279]
                tunnel: [w1274 w1278] -> w1268
                tunnel: w1267 -> [_ w1275]
                tunnel: w1266 -> [w1273 w1277]
                tunnel: [w1272 w1276] -> w1265
                frame False {
                  n556 = Insert Into Array(array=w1273, new element=0.0 ("Neues Element/Teil-Array")) -> (w1272:dbl[])  [unwired: 1 in]
                }
                frame True {
                  n557 = Insert Into Array(array=w1279, new element=w1275) -> (w1278:dbl[])  [unwired: 1 in]
                  n558 = Insert Into Array(array=w1277, new element=w1275) -> (w1276:dbl[])  [unwired: 1 in]
                }
              }
            }
            n559 = Index Array(array=w1158, index=3 ("Index")) -> (element=w1192:dbl)
            n560 = Index Array(array=w1158, index=0 ("Index")) -> (element=w1188:dbl)
            n561 = case shown="\"SISE chan #1\", Default" "?" {
              selector: "?" -> [w1234 w1244 w1252 w1260]
              tunnel: w1143 -> [w1239 w1246 w1256 w1263]
              tunnel: w1135 -> [w1240 w1247 w1255 w1264]
              tunnel: w1139 -> [w1236 w1243 w1250 w1259]
              tunnel: "Start fit (% of rec. period)" -> [w1238 w1245 w1254 w1262]
              frame "SISE chan #1", Default {
                n562 = Index Array(array=w1236, index=w1234) -> (element=w1235:bool)
                n563 = call "Feed-SISE-Probe-Graph.vi"("Boolesch"=w1235, "Numerisch"=2, "Array 2"=w1240, "Array"=w1239, "Start fit (% of rec. period)"=w1238) -> ("Array 3"=→"Vprobe SISE 1":cluster{dbl[], dbl[]}[])  [unwired: 6 in]
              }
              frame "SISE chan #2" {
                n564 = Index Array(array=w1243, index=w1244) -> (element=w1242:bool)
                n565 = call "Feed-SISE-Probe-Graph.vi"("Boolesch"=w1242, "Numerisch"=3, "Array 2"=w1247, "Array"=w1246, "Start fit (% of rec. period)"=w1245) -> ("Array 3"=→"Vprobe SISE 2":cluster{dbl[], dbl[]}[])  [unwired: 6 in]
              }
              frame "V chan #1" {
                n566 = Index Array(array=w1250, index=w1252) -> (element=w1251:bool)
                n567 = call "Feed-V-Probe-Graph.vi"("Boolesch"=w1251, "Numerisch"=4, "Array 2"=w1255, "Array"=w1256, "Start fit (% of rec. period)"=w1254) -> ("Array 3"=→"Vprobe V 1":cluster{dbl[], dbl[]}[])  [unwired: 6 in]
              }
              frame "V chan #2" {
                n568 = Index Array(array=w1259, index=w1260) -> (element=w1258:bool)
                n569 = call "Feed-V-Probe-Graph.vi"("Boolesch"=w1258, "Numerisch"=5, "Array 2"=w1264, "Array"=w1263, "Start fit (% of rec. period)"=w1262) -> ("Array 3"=→"Vprobe V 2":cluster{dbl[], dbl[]}[])  [unwired: 6 in]
              }
            }
            n570 = Divide(x=w1192, y=10.0) -> (x/y=w1187:dbl)
            n571 = case shown="1" w1127 {
              tunnel: w1197 -> [w1427 w1439 w1481 w1488 w1500 w1547]
              tunnel: w1199 -> [w1429 w1446 w1484 w1487 w1499 w1546]
              tunnel: [w1429 w1446 w1484 w1487 w1498 w1545] -> w1196
              tunnel: w1198 -> [_ w1445 _ _ _ _]
              tunnel: w1138 -> [_ w1433 _ _ w1492 w1539]
              tunnel: w1200 -> [w1428 w1432 w1480 w1486 w1495 w1542]
              tunnel: [w1428 w1432 w1480 w1486 w1496 w1543] -> w1122
              tunnel: [w1427 w1431 w1479 w1485 w1493 w1540] -> w1194
              tunnel: w1106 -> [_ w1430 _ _ _ _]
              frame 0, Default {
              }
              frame 1 {
                n572 = Index Array(array=w1445, index=0) -> (element=w1447:dbl)
                n573 = Index Array(array=w1445, index=1) -> (element=w1438:dbl)
                n574 = Cosine(x=w1438) -> (cos(x)=w1437:dbl)
                n575 = Sine(x=w1438) -> (sin(x)=w1436:dbl)
                n576 = Multiply(x=w1447, y=w1437) -> (x*y=w1444:dbl)
                n577 = Multiply(x=w1447, y=w1436) -> (x*y=w1443:dbl)
                n578 = Multiply(x=w1444, y=w1430) -> (x*y=w1441:dbl)
                n579 = Multiply(x=w1443, y=10.0) -> (x*y=w1442:dbl)
                n580 = for {
                  tunnel: w1446 -> [w1459] mode=indexing
                  tunnel: w1441 -> [w1461]
                  tunnel: w1442 -> [w1460]
                  shift-right: [w1455] -> w1435
                  shift-left: "ABS " -> [w1457]
                  tunnel: w1433 -> [w1450]
                  i -> [w1452]
                  n581 = case shown="True" w1450 {
                    tunnel: w1452 -> [w1462 _]
                    tunnel: [w1462 1] -> w1451
                    frame False {
                    }
                    frame True {
                    }
                  }
                  n582 = case shown="1" w1451 {
                    tunnel: w1461 -> [w1473 _ _]
                    tunnel: w1460 -> [_ _ w1477]
                    tunnel: w1459 -> [w1474 w1475 w1478]
                    tunnel: [w1472 w1475 w1476] -> w1458
                    frame 0, Default {
                      n583 = Add(x=w1474, y=w1473) -> (x+y=w1472:dbl)
                    }
                    frame 1 {
                    }
                    frame 2 {
                      n584 = Add(x=w1478, y=w1477) -> (x+y=w1476:dbl)
                    }
                  }
                  n585 = Number To Decimal String(number=w1458) -> (decimal integer string=w1456:string)  [unwired: 1 in]
                  n586 = Equal?(x=2, y=w1452) -> (x = y?=w1453:bool)
                  n587 = case shown="True" w1453 {
                    tunnel: w1457 -> [w1467 w1471]
                    tunnel: w1456 -> [w1466 w1469]
                    tunnel: [w1464 w1470] -> w1455
                    frame False {
                      n588 = Concatenate Strings(w1467, w1466, "\t") -> (w1464:string)
                    }
                    frame True {
                      n589 = Concatenate Strings(w1471, w1469, "\r\n") -> (w1470:string)
                    }
                  }
                }
                n590 = VISA Write(VISA resource name=w1439, write buffer=w1435) -> (VISA resource name out=w1431:refnum<visa-resource-name>)  [unwired: 1 in, 2 out]
              }
              frame 2 {
                n591 = property class="Instr"(reference=w1481) -> (reference out=w1482:refnum<visa-resource-name>, "Bytes at Port"=w1483:u32)  [unwired: 1 in, 1 out]
                n592 = VISA Read(VISA resource name=w1482, byte count=w1483) -> (VISA resource name out=w1479:refnum<visa-resource-name>)  [unwired: 1 in, 3 out]
              }
              frame 3 {
                n593 = Concatenate Strings("POS", "\r\n") -> (w1491:string)
                n594 = VISA Write(VISA resource name=w1488, write buffer=w1491) -> (VISA resource name out=w1485:refnum<visa-resource-name>)  [unwired: 1 in, 2 out]
              }
              frame 4 {
                n595 = property class="Instr"(reference=w1500) -> (reference out=w1502:refnum<visa-resource-name>, "Bytes at Port"=w1501:u32)  [unwired: 1 in, 1 out]
                n596 = VISA Read(VISA resource name=w1502, byte count=w1501) -> (VISA resource name out=w1494:refnum<visa-resource-name>, read buffer=w1497:string)  [unwired: 1 in, 2 out]
                n597 = case shown="True" w1492 {
                  tunnel: w1499 -> [w1518 w1537]
                  tunnel: [w1518 w1536] -> w1498
                  tunnel: w1497 -> [w1507 w1522]
                  tunnel: [w1512 w1531] -> w1496
                  tunnel: w1495 -> [w1511 w1530]
                  tunnel: w1494 -> [w1503 w1521]
                  tunnel: [w1503 w1521] -> w1493
                  frame False {
                    n598 = Match Pattern(string=w1511, regular expression="P0:") -> (match substring=w1516:string, after substring=w1515:string)  [unwired: 1 in, 2 out]
                    n599 = String Length(string=w1507) -> (length=w1510:i32)
                    n600 = Match Pattern(string=w1515, regular expression="P1:") -> (before substring=w1504:string, match substring=w1517:string)  [unwired: 1 in, 2 out]
                    n601 = Subtract(x=w1510, y=1) -> (x-y=w1508:i32)
                    n602 = String Subset(string=w1507, length (rest)=w1508) -> (substring=w1506:string)  [unwired: 1 in]
                    n603 = Concatenate Strings(w1516, w1504, w1517, w1506, "\t") -> (w1512:string)
                  }
                  frame True {
                    n604 = Match Pattern(string=w1530, regular expression="P0:") -> (match substring=w1532:string, after substring=w1534:string)  [unwired: 1 in, 2 out]
                    n605 = String Length(string=w1522) -> (length=w1529:i32)
                    n606 = Subtract(x=w1529, y=1) -> (x-y=w1527:i32)
                    n607 = Match Pattern(string=w1534, regular expression="P1:") -> (match substring=w1524:string, after substring=w1525:string)  [unwired: 1 in, 2 out]
                    n608 = String Subset(string=w1522, length (rest)=w1527) -> (substring=w1526:string)  [unwired: 1 in]
                    n609 = Concatenate Strings(w1532, w1526, "\t", w1524, w1525) -> (w1531:string)
                    n610 = call "GetAxisValuesI (SubVI).vi"("read buffer"=w1522) -> ("Array"=w1519:dbl[])  [unwired: 10 in]
                    n611 = Replace Array Subset(array=w1537, new element=w1519, index=0 ("Index")) -> (w1536:dbl[])
                  }
                }
              }
              frame 5 {
                n612 = property class="Instr"(reference=w1547) -> (reference out=w1549:refnum<visa-resource-name>, "Bytes at Port"=w1548:u32)  [unwired: 1 in, 1 out]
                n613 = VISA Read(VISA resource name=w1549, byte count=w1548) -> (VISA resource name out=w1541:refnum<visa-resource-name>, read buffer=w1544:string)  [unwired: 1 in, 2 out]
                n614 = case shown="True" w1539 {
                  tunnel: w1546 -> [w1565 w1584]
                  tunnel: [w1565 w1583] -> w1545
                  tunnel: w1544 -> [w1554 w1569]
                  tunnel: [w1559 w1578] -> w1543
                  tunnel: w1542 -> [w1558 w1577]
                  tunnel: w1541 -> [w1550 w1567]
                  tunnel: [w1550 w1566] -> w1540
                  tunnel: "Enable change position 0" -> [_ w1568]
                  frame False {
                    n615 = Match Pattern(string=w1558, regular expression="P0:") -> (match substring=w1563:string, after substring=w1562:string)  [unwired: 1 in, 2 out]
                    n616 = String Length(string=w1554) -> (length=w1557:i32)
                    n617 = Match Pattern(string=w1562, regular expression="P1:") -> (before substring=w1551:string, match substring=w1564:string)  [unwired: 1 in, 2 out]
                    n618 = Subtract(x=w1557, y=1) -> (x-y=w1555:i32)
                    n619 = String Subset(string=w1554, length (rest)=w1555) -> (substring=w1553:string)  [unwired: 1 in]
                    n620 = Concatenate Strings(w1563, w1551, w1564, w1553, "\t") -> (w1559:string)
                  }
                  frame True {
                    n621 = Match Pattern(string=w1577, regular expression="P0:") -> (match substring=w1579:string, after substring=w1581:string)  [unwired: 1 in, 2 out]
                    n622 = String Length(string=w1569) -> (length=w1576:i32)
                    n623 = Subtract(x=w1576, y=1) -> (x-y=w1574:i32)
                    n624 = Match Pattern(string=w1581, regular expression="P1:") -> (match substring=w1571:string, after substring=w1572:string)  [unwired: 1 in, 2 out]
                    n625 = String Subset(string=w1569, length (rest)=w1574) -> (substring=w1573:string)  [unwired: 1 in]
                    n626 = case shown="False" w1568 {
                      tunnel: w1584 -> [w1586 w1592]
                      tunnel: [w1586 w1591] -> w1583
                      tunnel: w1569 -> [_ w1590]
                      tunnel: w1567 -> [w1585 w1587]
                      tunnel: [w1585 w1587] -> w1566
                      frame False {
                      }
                      frame True {
                        n627 = call "GetAxisValuesI (SubVI).vi"("read buffer"=w1590) -> ("Array"=w1588:dbl[])  [unwired: 10 in]
                        n628 = Replace Array Subset(array=w1592, new element=w1588, index=0 ("Index")) -> (w1591:dbl[])
                      }
                    }
                    n629 = Concatenate Strings(w1579, w1573, "\t", w1571, w1572) -> (w1578:string)
                  }
                }
              }
            }
            n630 = case shown="True" w1177 {
              tunnel: w1122 -> [_ w1316]
              tunnel: [w1300 w1316] -> w1161
              tunnel: w1169 -> [w1301 _]
              tunnel: w1168 -> [w1296 w1325]
              tunnel: w1175 -> [w1299 w1324]
              tunnel: [w1298 w1316] -> w1159
              tunnel: w1176 -> [w1298 w1317]
              tunnel: [w1297 w1323] -> w1160
              frame False {
                n631 = case shown="True" w1301 {
                  tunnel: ["" "Event Mark"] -> w1300
                  tunnel: w1299 -> [_ w1315]
                  tunnel: w1296 -> [w1303 w1308]
                  tunnel: [w1303 w1309] -> w1297
                  frame False {
                  }
                  frame True {
                    n632 = Divide(x=w1315, y=60.0) -> (x/y=w1313:dbl)
                    n633 = Number To Fractional String(number=w1313, precision (6)=i16 2 ("Genauigkeit (6)")) -> (F-format string=w1311:string)  [unwired: 2 in]
                    n634 = Concatenate Strings(w1311, " min: ", "\t", "Event Mark", "\t") -> (w1307:string)
                    n635 = Insert Into Array(array=w1308, new element=w1307) -> (w1309:string[])  [unwired: 1 in]
                  }
                }
              }
              frame True {
                n636 = Match Pattern(string=w1316, regular expression="P1:") -> (before substring=w1320:string)  [unwired: 1 in, 3 out]
                n637 = Match Pattern(string=w1317, regular expression="P1:") -> (before substring=w1318:string)  [unwired: 1 in, 3 out]
                n638 = Not Equal?(x=w1320, y=w1318) -> (x != y?=w1322:bool)
                n639 = case shown="True" w1322 {
                  tunnel: w1325 -> [w1326 w1348]
                  tunnel: [w1326 w1349] -> w1323
                  tunnel: w1316 -> [_ w1337]
                  tunnel: w1317 -> [_ w1336]
                  tunnel: w1324 -> [_ w1334]
                  frame False {
                  }
                  frame True {
                    n640 = Divide(x=w1334, y=60.0) -> (x/y=w1332:dbl)
                    n641 = Match Pattern(string=w1337, regular expression="P0:") -> (after substring=w1347:string)  [unwired: 1 in, 3 out]
                    n642 = Number To Fractional String(number=w1332, precision (6)=i16 2) -> (F-format string=w1328:string)  [unwired: 2 in]
                    n643 = Match Pattern(string=w1336, regular expression="P0:") -> (after substring=w1342:string)  [unwired: 1 in, 3 out]
                    n644 = Match Pattern(string=w1347, regular expression="P1:") -> (before substring=w1346:string)  [unwired: 1 in, 3 out]
                    n645 = Match Pattern(string=w1342, regular expression="P1:") -> (before substring=w1341:string)  [unwired: 1 in, 3 out]
                    n646 = Concatenate Strings(w1328, "\t", "min: Move ") -> (w1331:string)
                    n647 = call "GetAxisValuesII (SubVI).vi"("read buffer"=w1346) -> ("Array"=w1343:dbl[])  [unwired: 10 in]
                    n648 = call "GetAxisValuesII (SubVI).vi"("read buffer"=w1341) -> ("Array"=w1338:dbl[])  [unwired: 10 in]
                    n649 = for {
                      tunnel: w1343 -> [w1359] mode=indexing
                      tunnel: w1338 -> [w1358] mode=indexing
                      shift-right: [w1360] -> w1329
                      shift-left: w1331 -> [w1361]
                      i -> [w1356]
                      n650 = Subtract(x=w1359, y=w1358) -> (x-y=w1353:dbl)
                      n651 = Divide(x=w1353, y=10.0) -> (x/y=w1355:dbl)
                      n652 = case shown="0, Default" w1356 {
                        tunnel: ["X " "Y " "Z "] -> w1352
                        frame 0, Default {
                        }
                        frame 1 {
                        }
                        frame 2 {
                        }
                      }
                      n653 = Number To Fractional String(number=w1355, precision (6)=i16 2 ("Genauigkeit (6)")) -> (F-format string=w1351:string)  [unwired: 2 in]
                      n654 = Concatenate Strings(w1361, w1352, w1351, "\t") -> (w1360:string)
                    }
                    n655 = Insert Into Array(array=w1348, new element=w1329) -> (w1349:string[])  [unwired: 1 in]
                  }
                }
              }
            }
            n656 = Greater?(x=w1187, y=w1137) -> (0:w1190:bool)
            n657 = case shown="True" w1190 {
              tunnel: w1188 -> [w1365 w1371]
              tunnel: w1137 -> [_ w1373]
              tunnel: w1138 -> [w1367 w1376]
              tunnel: w1187 -> [_ w1375]
              tunnel: [w1366 w1372] -> w1178
              tunnel: w1186 -> [_ w1370]
              frame False {
                n658 = case shown="False" w1367 {
                  tunnel: [w1368 0.0] -> w1366
                  tunnel: w1365 -> [w1368 _]
                  frame False {
                  }
                  frame True {
                  }
                }
              }
              frame True {
                n659 = Divide(x=w1371, y=w1375) -> (x/y=w1374:dbl)
                n660 = case shown="True" w1376 {
                  tunnel: w1373 -> [w1379 w1383]
                  tunnel: w1374 -> [w1378 w1387]
                  tunnel: [w1377 w1381] -> w1372
                  tunnel: w1371 -> [_ w1386]
                  tunnel: w1370 -> [_ w1380]
                  frame False {
                    n661 = Multiply(x=w1378, y=w1379) -> (x*y=w1377:dbl)
                  }
                  frame True {
                    n662 = Multiply(x=w1387, y=w1383) -> (x*y=w1388:dbl)
                    n663 = Equal?(x=w1380, y=0) -> (x = y?=w1385:bool)
                    n664 = Subtract(x=w1386, y=w1388) -> (x-y=w1382:dbl)
                    n665 = case shown="True" w1385 {
                      tunnel: [w1389 0.0] -> w1381
                      tunnel: w1382 -> [w1389 _]
                      frame False {
                      }
                      frame True {
                      }
                    }
                  }
                }
              }
            }
            n666 = Build Array(w1175, w1178) -> (w1123:dbl[])
            n667 = call "EsingleGenerator.vi"("Numeric in"=w1137, "Boolean"=w1138) -> ("Numeric out"=w1134:dbl)  [unwired: 9 in]
            n668 = Random Number (0-1)() -> (number: 0 to 1=w1151:dbl)
            n669 = Random Number (0-1)() -> (number: 0 to 1=w1182:dbl)
            n670 = Add(x=w1134, y=6.0) -> (x+y=w1150:dbl)
            n671 = Add(x=w1134, y=8.0) -> (x+y=w1181:dbl)
            n672 = Insert Into Array(array=w1123, new element=w1124) -> (w1125:dbl[])  [unwired: 1 in]
            n673 = Insert Into Array(array=w1123, new element=w1132) -> (w1130:dbl[])  [unwired: 1 in]
            n674 = for {
              tunnel: w1130 -> [w1230] mode=indexing
              shift-right: [w1229] -> w1129
              shift-left: "" -> [w1231]
              n675 = Number To Fractional String(number=w1230) -> (F-format string=w1232:string)  [unwired: 3 in]
              n676 = Concatenate Strings(w1231, w1232, "\t") -> (w1229:string)
            }
            n677 = Add(x=w1150, y=w1151) -> (x+y=w1147:dbl)
            n678 = Add(x=w1181, y=w1182) -> (x+y=w1148:dbl)
            n679 = case shown="False" "Stop measurent" {
              tunnel: [w1593 TRUE] -> w1121
              tunnel: w1217 -> [w1593 _]
              frame False {
              }
              frame True {
              }
            }
            "Stop recording" <- w1121
            n680 = Build Array(w1148, w1147, -10.0, -20.0) -> ()  [unwired: 1 out]
            n681 = Insert Into Array(array=w1135, new element=w1125) -> (w1141:dbl[][])  [unwired: 2 in]
            n682 = Concatenate Strings(w1129, w1161, "\r\n") -> (w1162:string)
            n683 = Write to Text File(file (use dialog)=w1165, text=w1162, error in=w1166) -> (refnum out=w1164:refnum<file>, error out=w1163:errorcluster)  [unwired: 1 in, 1 out]
          }
          "Stop recording 2" <- w1057
          n684 = Bundle(w1063, w1075) -> (w1074:cluster{string[], dbl[][]})  [unwired: 1 in]
          n685 = Enqueue Element(queue=w1080, element=w1074, error in (no error)=w1079) -> (queue out=w1078:refnum<queue>, error out=w1077:errorcluster)  [unwired: 1 in, 1 out]
        }
        n686 = Unbundle(w513) -> ("status"=w550:bool, "code"=w549:i32, "source"=w548:string)
        n687 = call <vilib>:"DAQmx Stop Task.vi"("task/channels in"=w514, "error in"=w513) -> ()  [unwired: 12 in, 2 out]
        n688 = Close File(refnum=w511, error in=w512) -> ()  [unwired: 2 out]
        n689 = Unbundle(w512) -> ("status"=w529:bool, "code"=w528:i32, "source"=w527:string)
        n690 = Bundle("task out"=w514, "status"=w550, "code"=w549, "source"=w548) -> (w547:T5)  [unwired: 1 in]
        n691 = Bundle("refnum out"=w511, "status"=w529, "code"=w528, "source"=w527) -> (w526:T4)  [unwired: 1 in]
        n692 = Release Queue(queue=w545, error in (no error)=w544) -> ()  [unwired: 1 in, 3 out]
      }
      frame 2 {
        n693 = while {
          tunnel: w1597 -> [w1605]
          tunnel: [w1604] -> w1596
          stop <- w1608 stop-if-true
          n694 = Wait (ms)(milliseconds to wait=u32 100 ("Zu wartende ms")) -> ()  [unwired: 1 out]
          n695 = case shown="True" "Stop programm" {
            tunnel: w1605 -> [w1610 _]
            tunnel: [w1610 TRUE] -> w1604
            frame False {
            }
            frame True {
            }
          }
          n696 = Or(x="New measurement", y="Stop programm") -> (x .or. y?=w1608:bool)
        }
      }
    }
    "Registerkarte" <- w27
  }
